vi "Adquisicion_6218.vi"() -> ()   [LabVIEW 2011]
uses:
  <vilib>/Utility/config.llb/Read Key (String).vi
  <vilib>/Utility/config.llb/Read Key (Double).vi
  <vilib>/Utility/config.llb/Write Key (String).vi
  <vilib>/Utility/config.llb/Write Key (Double).vi
  <vilib>/Utility/config.llb/NI_LVConfig.lvlib
  <vilib>/Analysis/NI_AALBase.lvlib
panel:
  out "Boolean 10":bool
  in  "Guardar":bool
  in  "Path2":bool
  in  "Datapath":bool
  in  "Path1":bool=TRUE
  in  "Tiempo":dbl
  in  "index 3":i32
  in  "index":i32
  out "reset3":bool
  out "reset2":bool
  out "reset":bool
  out "Time has Elapsed 2":bool caption="Time has Elapsed"
  out "Time has Elapsed":bool
  out "appended array":string[](array[string])
  in  "Tab Control 9":enum32{"Page 1", "Page 2", "Page 3"}(tab)
  in  "CH16":string="CH16"
  in  "CH15":string="CH15"
  in  "CH14":string="CH14"
  in  "CH13":string="CH13"
  in  "CH12":string="CH12"
  in  "CH11":string="CH11"
  in  "CH10":string="CH10"
  in  "CH9":string="CH9"
  in  "Tasa de Adquisicion":dbl=1000.0
  in  "CH8":string="CH8"
  in  "CH7":string="CH7"
  in  "CH6":string="CH6"
  in  "CH5":string="CH5"
  in  "CH4 2":string="CH4"
  in  "CH3":string="CH3"
  in  "CH2 2":string="CH2"
  in  "CH1":string="CH1"
  out "Voltaje":dbl
  out "Medida":dbl
  in  "m1":dbl
  in  "b1":dbl
  out "Voltaje":dbl
  in  "m2":dbl
  in  "b2":dbl
  out "Medida":dbl
  in  "m3":dbl
  in  "m4":dbl
  in  "b3":dbl
  in  "b4":dbl
  out "Voltaje":dbl
  out "Voltaje":dbl
  out "Medida":dbl
  out "Medida":dbl
  out "Medida":dbl
  in  "b5":dbl
  in  "m5":dbl
  out "Voltaje":dbl
  out "Medida":dbl
  in  "m6":dbl
  in  "b6":dbl
  out "Voltaje":dbl
  out "Medida":dbl
  in  "m7":dbl
  in  "b7":dbl
  out "Voltaje":dbl
  out "Voltaje":dbl
  in  "b8":dbl
  in  "m8":dbl
  out "Medida":dbl
  out "CH1":string
  out "CH2":string
  out "CH3":string
  out "CH4":string
  out "CH5":string
  out "CH6":string
  out "CH7":string
  out "CH8":string
  in  "Boolean":bool=TRUE
  in  "Boolean 2":bool=TRUE
  in  "Boolean 3":bool=TRUE
  in  "Boolean 4":bool=TRUE
  in  "Boolean 6":bool=TRUE
  in  "Boolean 5":bool=TRUE
  in  "Boolean 7":bool=TRUE
  in  "Boolean 8":bool=TRUE
  in  "Numero de Muestras":i32=1
  in  "file path":path=path "C:/Users/Zulueta/Documents/Pasantia/Mediciones"
  out "Tiempo":dbl caption="Elapsed Time (s)"
  in  "Iniciar":bool
  out "Boolean 9":bool
  in  "reset 2":bool caption="reset"
  out "q'":bool
  out "Tiempo":dbl caption="Elapsed Time (s)"
  in  "file path 2":path=path "C:/Users/Zulueta/Documents/Pasantia/Mediciones_Tiempo"
  out "Tiempo":dbl caption="Elapsed Time (s)"
  out "q2'":bool
  in  "?":bool
  in  "file path 3":path=path "C:/Users/Zulueta/Documents/Pasantia/Mediciones_Promedio"
  in  "Tiempo \nde adquisición":enum32{"Segundos", "Minutos", "Horas"}(tab) caption="Tiempo de adquisición"
  in  "?":dbl
  in  "?":dbl
  in  "?":dbl
  in  "stop":bool
  in  "Guardar Configuracion":bool
  in  "s":bool=TRUE
  in  "m9":dbl
  in  "b9":dbl
  out "s? t:f":dbl
  out "x+y":dbl
  in  "s 3":bool=TRUE
  out "s? t:f 2":dbl
  in  "m10":dbl
  in  "b10":dbl
  out "x+y 2":dbl
  out "s? t:f 3":dbl
  in  "m11":dbl
  in  "b11":dbl
  in  "s 6":bool=TRUE
  out "x+y 3":dbl
  in  "s 7":bool=TRUE
  out "s? t:f 4":dbl
  in  "m12":dbl
  in  "b12":dbl
  out "x+y 4":dbl
  in  "s 9":bool=TRUE
  in  "m13":dbl
  out "s? t:f 5":dbl
  in  "b13":dbl
  out "x+y 5":dbl
  in  "m14":dbl
  out "s? t:f 6":dbl
  in  "s 11":bool=TRUE
  in  "b14":dbl
  out "x+y 6":dbl
  in  "s 13":bool=TRUE
  out "s? t:f 7":dbl
  in  "m15":dbl
  in  "b15":dbl
  out "x+y 7":dbl
  in  "s 15":bool=TRUE
  in  "m16":dbl
  out "x+y 8":dbl
  out "s? t:f 8":dbl
  in  "b16":dbl
  out "CH9":string="CH8"
  out "CH10":string="CH10"
  out "CH11":string="CH11"
  out "CH12":string="CH12"
  out "CH13 3":string="CH13"
  out "CH14 3":string="CH14"
  out "CH15 3":string="CH15"
  out "CH16 3":string="CH16"
  out "Waveform Chart 17":dbl(graph)
  out "Waveform Chart 16":dbl(graph)
  out "Waveform Chart 15":dbl(graph)
  out "Waveform Chart 14":dbl(graph)
  out "Waveform Chart 13":dbl(graph)
  out "Waveform Chart 12":dbl(graph)
  out "Waveform Chart 11":dbl(graph)
  out "Waveform Chart 2":dbl(graph)
  out "Waveform Chart 10":dbl(graph)
  out "Waveform Chart 9":dbl(graph)
  out "Waveform Chart 8":dbl(graph)
  out "Waveform Chart 7":dbl(graph)
  out "Waveform Chart 6":dbl(graph)
  out "Waveform Chart 5":dbl(graph)
  out "Waveform Chart 4":dbl(graph)
  out "Waveform Chart 3":dbl(graph)
  out "CH1":string
  out "CH2":string
  out "CH3":string
  out "CH4":string
  out "CH5":string
  out "CH6":string
  out "CH7":string
  out "CH8":string
  in  "Boolean 18":bool=TRUE
  in  "Boolean 19":bool=TRUE
  in  "Boolean 20":bool=TRUE
  in  "Boolean 21":bool=TRUE
  in  "Boolean 22":bool=TRUE
  in  "Boolean 23":bool=TRUE
  in  "Boolean 24":bool=TRUE
  in  "Boolean 25":bool=TRUE
  in  "s 2":bool=TRUE
  in  "s 4":bool
  in  "s 5":bool
  in  "s 8":bool
  in  "s 10":bool
  in  "s 12":bool
  in  "s 14":bool
  in  "s 16":bool
  out "CH9 3":string="CH8"
  out "CH10 2":string="CH8"
  out "CH11 2":string="CH8"
  out "CH12 2":string="CH8"
  out "CH13 2":string="CH8"
  out "CH14 2":string="CH8"
  out "CH15 2":string="CH8"
  out "CH16 2":string="CH8"
  out "Waveform Chart":T1(graph)
  out "Time":dbl
  # "On/Off"
  # "Pendiente"
  # "Medida"
  # "Offset"
  # "Voltaje"
  # "Aquirir muestras por solicitud"
  # "Adquirir muestras por tiempo definido"
  # "Adquirir promedio de cada canal en un tiempo T"
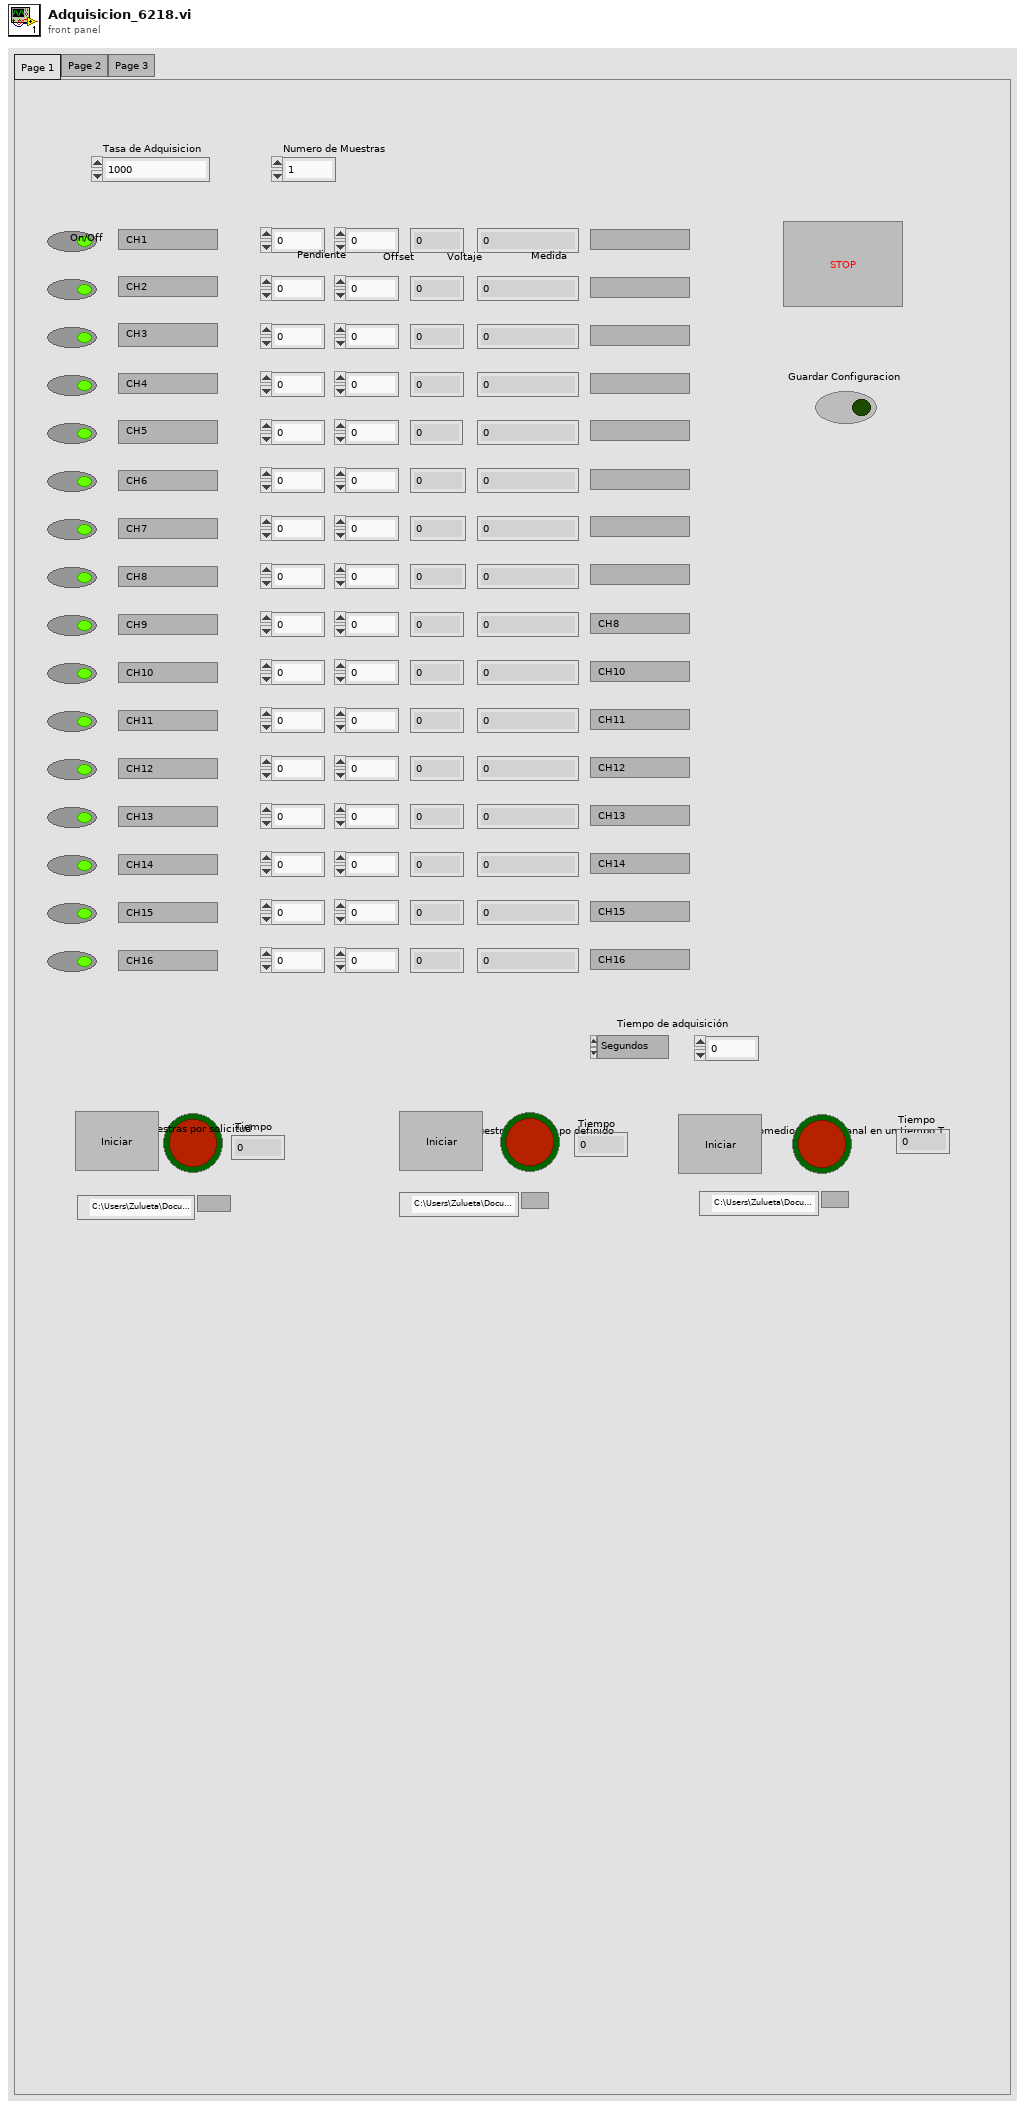
[diagram p1: front panel]
types:
  T1 = cluster{dbl, dbl, dbl, dbl, dbl, dbl, dbl, dbl, dbl, dbl, dbl, dbl, dbl, dbl, dbl, dbl}
  T2 = enum16{"big-endian, network order", "native, host order", "little-endian"}
  T3 = enum16{"open", "open or create", "create or replace", "create", "open (read-only)"}
  T4 = typedef "NI_LVConfig.lvlib/Config Data RefNum.ctl" = refnum<k1>
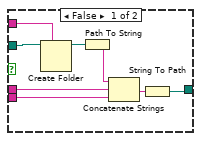
[diagram p2: hidden frame]
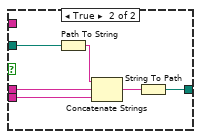
[diagram p3: hidden frame]
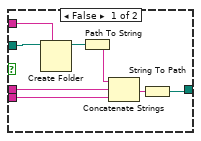
[diagram p4: hidden frame]
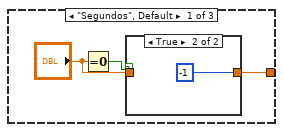
[diagram p11: hidden frame]
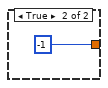
[diagram p13: hidden frame]
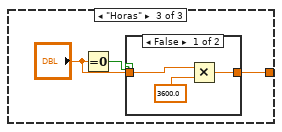
[diagram p14: hidden frame]
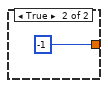
[diagram p15: hidden frame]
diagram:
  w177 = "_" ("replace string (\"\")")
  w178 = ":" ("search string")
  w110 = "\\" ("string")
  w156 = 0.0
  w6 = "Offsets" ("section")
  w44 = "Pendientes" ("section")
  w83 = TRUE ("read raw string? (F)")
  w74 = "Nombres_Canales" ("section")
  n1 = call <vilib>:"Open Config Data.vi"("configuration file path"=path "C:/Users/Zulueta/Documents/Pasantia/Configuracion_16Canales") -> ("error out"=w306:errorcluster, "refnum"=w307:T4)  [unwired: 8 in, 1 out]
  n2 = call-poly <vilib>:"Read Key.vi"("read raw string? (F)"=w83, "section"=w74, "error in (no error)"=w306, "key"="C1", "refnum"=w307) -> ("error out"=w302:errorcluster, "value"=w309:string, "refnum out"=w303:T4)  [unwired: 3 in, 1 out]
  n3 = property on="CH1" class="Str"("Value"=w309) -> ()  [unwired: 2 in, 2 out]
  n4 = call-poly <vilib>:"Read Key.vi"("read raw string? (F)"=w83, "section"=w74, "error in (no error)"=w302, "key"="C2", "refnum"=w303) -> ("error out"=w299:errorcluster, "value"=w304:string, "refnum out"=w298:T4)  [unwired: 3 in, 1 out]
  n5 = property on="CH2 2" class="Str"("Value"=w304) -> ()  [unwired: 2 in, 2 out]
  n6 = call-poly <vilib>:"Read Key.vi"("read raw string? (F)"=w83, "section"=w74, "error in (no error)"=w299, "key"="C3", "refnum"=w298) -> ("error out"=w295:errorcluster, "value"=w301:string, "refnum out"=w296:T4)  [unwired: 3 in, 1 out]
  n7 = property on="CH3" class="Str"("Value"=w301) -> ()  [unwired: 2 in, 2 out]
  n8 = call-poly <vilib>:"Read Key.vi"("read raw string? (F)"=w83, "section"=w74, "error in (no error)"=w295, "key"="C4", "refnum"=w296) -> ("error out"=w292:errorcluster, "value"=w297:string, "refnum out"=w293:T4)  [unwired: 3 in, 1 out]
  n9 = property on="CH4 2" class="Str"("Value"=w297) -> ()  [unwired: 2 in, 2 out]
  n10 = call-poly <vilib>:"Read Key.vi"("read raw string? (F)"=w83, "section"=w74, "error in (no error)"=w292, "key"="C5", "refnum"=w293) -> ("error out"=w287:errorcluster, "value"=w290:string, "refnum out"=w288:T4)  [unwired: 3 in, 1 out]
  n11 = property on="CH5" class="Str"("Value"=w290) -> ()  [unwired: 2 in, 2 out]
  n12 = call-poly <vilib>:"Read Key.vi"("read raw string? (F)"=w83, "section"=w74, "error in (no error)"=w287, "key"="C6", "refnum"=w288) -> ("error out"=w284:errorcluster, "value"=w289:string, "refnum out"=w285:T4)  [unwired: 3 in, 1 out]
  n13 = property on="CH6" class="Str"("Value"=w289) -> ()  [unwired: 2 in, 2 out]
  n14 = call-poly <vilib>:"Read Key.vi"("read raw string? (F)"=w83, "section"=w74, "error in (no error)"=w284, "key"="C7", "refnum"=w285) -> ("error out"=w279:errorcluster, "value"=w283:string, "refnum out"=w280:T4)  [unwired: 3 in, 1 out]
  n15 = property on="CH7" class="Str"("Value"=w283) -> ()  [unwired: 2 in, 2 out]
  n16 = call-poly <vilib>:"Read Key.vi"("read raw string? (F)"=w83, "section"=w74, "error in (no error)"=w279, "key"="C8", "refnum"=w280) -> ("error out"=w105:errorcluster, "value"=w281:string, "refnum out"=w106:T4)  [unwired: 3 in, 1 out]
  n17 = property on="CH8" class="Str"("Value"=w281) -> ()  [unwired: 2 in, 2 out]
  n18 = call-poly <vilib>:"Read Key.vi"("read raw string? (F)"=w83, "section"=w74, "error in (no error)"=w105, "key"="C9", "refnum"=w106) -> ("error out"=w101:errorcluster, "value"=w103:string, "refnum out"=w102:T4)  [unwired: 3 in, 1 out]
  n19 = property on="CH9" class="Str"("Value"=w103) -> ()  [unwired: 2 in, 2 out]
  n20 = call-poly <vilib>:"Read Key.vi"("read raw string? (F)"=w83, "section"=w74, "error in (no error)"=w101, "key"="C10", "refnum"=w102) -> ("error out"=w98:errorcluster, "value"=w97:string, "refnum out"=w99:T4)  [unwired: 3 in, 1 out]
  n21 = property on="CH10" class="Str"("Value"=w97) -> ()  [unwired: 2 in, 2 out]
  n22 = call-poly <vilib>:"Read Key.vi"("read raw string? (F)"=w83, "section"=w74, "error in (no error)"=w98, "key"="C11", "refnum"=w99) -> ("error out"=w93:errorcluster, "value"=w95:string, "refnum out"=w94:T4)  [unwired: 3 in, 1 out]
  n23 = property on="CH11" class="Str"("Value"=w95) -> ()  [unwired: 2 in, 2 out]
  n24 = call-poly <vilib>:"Read Key.vi"("read raw string? (F)"=w83, "section"=w74, "error in (no error)"=w93, "key"="C12", "refnum"=w94) -> ("error out"=w89:errorcluster, "value"=w91:string, "refnum out"=w90:T4)  [unwired: 3 in, 1 out]
  n25 = property on="CH12" class="Str"("Value"=w91) -> ()  [unwired: 2 in, 2 out]
  n26 = call-poly <vilib>:"Read Key.vi"("read raw string? (F)"=w83, "section"=w74, "error in (no error)"=w89, "key"="C13", "refnum"=w90) -> ("error out"=w86:errorcluster, "value"=w85:string, "refnum out"=w87:T4)  [unwired: 3 in, 1 out]
  n27 = property on="CH13" class="Str"("Value"=w85) -> ()  [unwired: 2 in, 2 out]
  n28 = call-poly <vilib>:"Read Key.vi"("read raw string? (F)"=w83, "section"=w74, "error in (no error)"=w86, "key"="C14", "refnum"=w87) -> ("error out"=w81:errorcluster, "value"=w79:string, "refnum out"=w82:T4)  [unwired: 3 in, 1 out]
  n29 = property on="CH14" class="Str"("Value"=w79) -> ()  [unwired: 2 in, 2 out]
  n30 = call-poly <vilib>:"Read Key.vi"("section"=w74, "error in (no error)"=w81, "key"="C15", "refnum"=w82) -> ("error out"=w77:errorcluster, "value"=w78:string, "refnum out"=w76:T4)  [unwired: 4 in, 1 out]
  n31 = Obtain Queue(name (unnamed)="CH9", element data type=w156) -> (queue out=w137:refnum<queue>)  [unwired: 3 in, 2 out]
  n32 = Obtain Queue(name (unnamed)="CH9(PSI)", element data type=w156) -> (queue out=w136:refnum<queue>)  [unwired: 3 in, 2 out]
  n33 = Obtain Queue(name (unnamed)="CH10", element data type=w156) -> (queue out=w135:refnum<queue>)  [unwired: 3 in, 2 out]
  n34 = Obtain Queue(name (unnamed)="CH1", element data type=w156) -> (queue out=w153:refnum<queue>)  [unwired: 3 in, 2 out]
  n35 = Obtain Queue(name (unnamed)="CH1(PSI)", element data type=w156) -> (queue out=w152:refnum<queue>)  [unwired: 3 in, 2 out]
  n36 = Obtain Queue(name (unnamed)="CH2", element data type=w156) -> (queue out=w151:refnum<queue>)  [unwired: 3 in, 2 out]
  n37 = Obtain Queue(name (unnamed)="CH2(PSI)", element data type=w156) -> (queue out=w150:refnum<queue>)  [unwired: 3 in, 2 out]
  n38 = Obtain Queue(name (unnamed)="CH3", element data type=w156) -> (queue out=w149:refnum<queue>)  [unwired: 3 in, 2 out]
  n39 = Obtain Queue(name (unnamed)="CH3(PSI)", element data type=w156) -> (queue out=w148:refnum<queue>)  [unwired: 3 in, 2 out]
  n40 = Obtain Queue(name (unnamed)="CH4", element data type=w156) -> (queue out=w147:refnum<queue>)  [unwired: 3 in, 2 out]
  n41 = Obtain Queue(name (unnamed)="CH4(PSI)", element data type=w156) -> (queue out=w146:refnum<queue>)  [unwired: 3 in, 2 out]
  n42 = Obtain Queue(name (unnamed)="CH5", element data type=w156) -> (queue out=w145:refnum<queue>)  [unwired: 3 in, 2 out]
  n43 = Obtain Queue(name (unnamed)="CH5(PSI)", element data type=w156) -> (queue out=w144:refnum<queue>)  [unwired: 3 in, 2 out]
  n44 = Obtain Queue(name (unnamed)="CH6", element data type=w156) -> (queue out=w143:refnum<queue>)  [unwired: 3 in, 2 out]
  n45 = Obtain Queue(name (unnamed)="CH6(PSI)", element data type=w156) -> (queue out=w142:refnum<queue>)  [unwired: 3 in, 2 out]
  n46 = Obtain Queue(name (unnamed)="CH7", element data type=w156) -> (queue out=w141:refnum<queue>)  [unwired: 3 in, 2 out]
  n47 = Obtain Queue(name (unnamed)="CH7(PSI)", element data type=w156) -> (queue out=w140:refnum<queue>)  [unwired: 3 in, 2 out]
  n48 = Obtain Queue(name (unnamed)="CH8", element data type=w156) -> (queue out=w139:refnum<queue>)  [unwired: 3 in, 2 out]
  n49 = Obtain Queue(name (unnamed)="CH8(PSI)", element data type=w156) -> (queue out=w138:refnum<queue>)  [unwired: 3 in, 2 out]
  n50 = Obtain Queue(name (unnamed)="CH10(PSI)", element data type=w156) -> (queue out=w134:refnum<queue>)  [unwired: 3 in, 2 out]
  n51 = Obtain Queue(name (unnamed)="CH11", element data type=w156) -> (queue out=w133:refnum<queue>)  [unwired: 3 in, 2 out]
  n52 = Obtain Queue(name (unnamed)="CH11(PSI)", element data type=w156) -> (queue out=w132:refnum<queue>)  [unwired: 3 in, 2 out]
  n53 = Obtain Queue(name (unnamed)="CH12", element data type=w156) -> (queue out=w131:refnum<queue>)  [unwired: 3 in, 2 out]
  n54 = Obtain Queue(name (unnamed)="CH12(PSI)", element data type=w156) -> (queue out=w130:refnum<queue>)  [unwired: 3 in, 2 out]
  n55 = Obtain Queue(name (unnamed)="CH13", element data type=w156) -> (queue out=w129:refnum<queue>)  [unwired: 3 in, 2 out]
  n56 = Obtain Queue(name (unnamed)="CH13(PSI)", element data type=w156) -> (queue out=w128:refnum<queue>)  [unwired: 3 in, 2 out]
  n57 = Obtain Queue(name (unnamed)="CH14", element data type=w156) -> (queue out=w127:refnum<queue>)  [unwired: 3 in, 2 out]
  n58 = Obtain Queue(name (unnamed)="CH14(PSI)", element data type=w156) -> (queue out=w126:refnum<queue>)  [unwired: 3 in, 2 out]
  n59 = Obtain Queue(name (unnamed)="CH15", element data type=w156) -> (queue out=w125:refnum<queue>)  [unwired: 3 in, 2 out]
  n60 = Obtain Queue(name (unnamed)="CH15(PSI)", element data type=w156) -> (queue out=w124:refnum<queue>)  [unwired: 3 in, 2 out]
  n61 = Obtain Queue(name (unnamed)="CH16", element data type=w156) -> (queue out=w123:refnum<queue>)  [unwired: 3 in, 2 out]
  n62 = Obtain Queue(name (unnamed)="CH16(PSI)", element data type=w156) -> (queue out=w122:refnum<queue>)  [unwired: 3 in, 2 out]
  n63 = property on="CH15" class="Str"("Value"=w78) -> ()  [unwired: 2 in, 2 out]
  n64 = call-poly <vilib>:"Read Key.vi"("section"=w74, "error in (no error)"=w77, "key"="C16", "refnum"=w76) -> ("error out"=w72:errorcluster, "value"=w71:string, "refnum out"=w73:T4)  [unwired: 4 in, 1 out]
  n65 = property on="CH16" class="Str"("Value"=w71) -> ()  [unwired: 2 in, 2 out]
  n66 = call-poly <vilib>:"Read Key.vi"("section"=w44, "error in (no error)"=w72, "key"="M1", "refnum"=w73) -> ("error out"=w274:errorcluster, "value"=w277:dbl, "refnum out"=w275:T4)  [unwired: 4 in, 1 out]
  n67 = property on="m1" class="DigNum (strict)"("Value"=w277) -> ()  [unwired: 2 in, 2 out]
  n68 = call-poly <vilib>:"Read Key.vi"("section"=w44, "error in (no error)"=w274, "key"="M2", "refnum"=w275) -> ("error out"=w270:errorcluster, "value"=w273:dbl, "refnum out"=w271:T4)  [unwired: 4 in, 1 out]
  n69 = property on="m2" class="DigNum (strict)"("Value"=w273) -> ()  [unwired: 2 in, 2 out]
  n70 = call-poly <vilib>:"Read Key.vi"("section"=w44, "error in (no error)"=w270, "key"="M3", "refnum"=w271) -> ("error out"=w267:errorcluster, "value"=w269:dbl, "refnum out"=w266:T4)  [unwired: 4 in, 1 out]
  n71 = property on="m3" class="DigNum (strict)"("Value"=w269) -> ()  [unwired: 2 in, 2 out]
  n72 = call-poly <vilib>:"Read Key.vi"("section"=w44, "error in (no error)"=w267, "key"="M4", "refnum"=w266) -> ("error out"=w263:errorcluster, "value"=w265:dbl, "refnum out"=w262:T4)  [unwired: 4 in, 1 out]
  n73 = property on="m4" class="DigNum (strict)"("Value"=w265) -> ()  [unwired: 2 in, 2 out]
  n74 = call-poly <vilib>:"Read Key.vi"("section"=w44, "error in (no error)"=w263, "key"="M5", "refnum"=w262) -> ("error out"=w259:errorcluster, "value"=w261:dbl, "refnum out"=w258:T4)  [unwired: 4 in, 1 out]
  n75 = property on="m5" class="DigNum (strict)"("Value"=w261) -> ()  [unwired: 2 in, 2 out]
  n76 = call-poly <vilib>:"Read Key.vi"("section"=w44, "error in (no error)"=w259, "key"="M6", "refnum"=w258) -> ("error out"=w254:errorcluster, "value"=w257:dbl, "refnum out"=w255:T4)  [unwired: 4 in, 1 out]
  n77 = property on="m6" class="DigNum (strict)"("Value"=w257) -> ()  [unwired: 2 in, 2 out]
  n78 = call-poly <vilib>:"Read Key.vi"("section"=w44, "error in (no error)"=w254, "key"="M7", "refnum"=w255) -> ("error out"=w251:errorcluster, "value"=w253:dbl, "refnum out"=w250:T4)  [unwired: 4 in, 1 out]
  n79 = property on="m7" class="DigNum (strict)"("Value"=w253) -> ()  [unwired: 2 in, 2 out]
  n80 = while {
    tunnel: w153 -> [w421]
    tunnel: w151 -> [w516]
    tunnel: w149 -> [w515]
    tunnel: w147 -> [w514]
    tunnel: w145 -> [w513]
    tunnel: w143 -> [w512]
    tunnel: w141 -> [w511]
    tunnel: w139 -> [w510]
    tunnel: w152 -> [w506]
    tunnel: w150 -> [w501]
    tunnel: w148 -> [w500]
    tunnel: w146 -> [w495]
    tunnel: w142 -> [w485]
    tunnel: w144 -> [w490]
    tunnel: w140 -> [w484]
    tunnel: w138 -> [w483]
    shift-right: [w420] -> _
    shift-left: w156 -> [w320]
    tunnel: w137 -> [w414]
    tunnel: w136 -> [w406]
    tunnel: w135 -> [w402]
    tunnel: w134 -> [w394]
    tunnel: w133 -> [w390]
    tunnel: w132 -> [w387]
    tunnel: w131 -> [w378]
    tunnel: w130 -> [w377]
    tunnel: w129 -> [w367]
    tunnel: w128 -> [w365]
    tunnel: w127 -> [w355]
    tunnel: w126 -> [w354]
    tunnel: w125 -> [w342]
    tunnel: w124 -> [w341]
    tunnel: w123 -> [w330]
    tunnel: w122 -> [w328]
    stop <- "stop" stop-if-true
    w329 = 0.0 ("f")
    n81 = call "DAQ Assistant"("rate"="Tasa de Adquisicion", "number of samples"="Numero de Muestras") -> ("data"=w417:dynamicdata, "error out"=w418:errorcluster)  [unwired: 14 in, 2 out]
    n82 = call <vilib>:"Clear Errors.vi"("error in (no error)"=w418) -> ()  [unwired: 6 in, 1 out]
    n83 = Split Signals(w417) -> (w469:dynamicdata, w504:dynamicdata, w499:dynamicdata, w494:dynamicdata, w489:dynamicdata, w482:dynamicdata, w478:dynamicdata, w474:dynamicdata, w411:dynamicdata, w401:dynamicdata, w381:dynamicdata, w375:dynamicdata, w352:dynamicdata, w338:dynamicdata, w339:dynamicdata, w326:dynamicdata)  [unwired: 16 in]
    n84 = call "Convert from Dynamic Data"("Dynamic Data Type"=w469) -> ("Scalar"=w458:dbl)  [unwired: 3 in]
    n85 = call "Convert from Dynamic Data2"("Dynamic Data Type"=w504) -> ("Scalar"=w468:dbl)  [unwired: 3 in]
    n86 = call "Convert from Dynamic Data3"("Dynamic Data Type"=w499) -> ("Scalar"=w466:dbl)  [unwired: 3 in]
    n87 = call "Convert from Dynamic Data4"("Dynamic Data Type"=w494) -> ("Scalar"=w464:dbl)  [unwired: 3 in]
    n88 = call "Convert from Dynamic Data5"("Dynamic Data Type"=w489) -> ("Scalar"=w462:dbl)  [unwired: 3 in]
    n89 = Select(t=w458, s="Boolean", f=w329) -> (s? t:f=w457:dbl)
    "Voltaje" <- w457
    n90 = call "Convert from Dynamic Data6"("Dynamic Data Type"=w482) -> ("Scalar"=w460:dbl)  [unwired: 3 in]
    n91 = call "Convert from Dynamic Data7"("Dynamic Data Type"=w478) -> ("Scalar"=w450:dbl)  [unwired: 3 in]
    n92 = call "Convert from Dynamic Data11"("Dynamic Data Type"=w381) -> ("Scalar"=w382:dbl)  [unwired: 3 in]
    n93 = call "Convert from Dynamic Data12"("Dynamic Data Type"=w375) -> ("Scalar"=w376:dbl)  [unwired: 3 in]
    n94 = call "Convert from Dynamic Data13"("Dynamic Data Type"=w352) -> ("Scalar"=w364:dbl)  [unwired: 3 in]
    n95 = call "Convert from Dynamic Data14"("Dynamic Data Type"=w338) -> ("Scalar"=w353:dbl)  [unwired: 3 in]
    n96 = call "Convert from Dynamic Data9"("Dynamic Data Type"=w411) -> ("Scalar"=w412:dbl)  [unwired: 3 in]
    n97 = call "Convert from Dynamic Data10"("Dynamic Data Type"=w401) -> ("Scalar"=w400:dbl)  [unwired: 3 in]
    n98 = call "Convert from Dynamic Data15"("Dynamic Data Type"=w339) -> ("Scalar"=w340:dbl)  [unwired: 3 in]
    n99 = Select(t=w468, s="Boolean 2", f=w329) -> (s? t:f=w456:dbl)
    "Voltaje" <- w456
    n100 = call "Convert from Dynamic Data8"("Dynamic Data Type"=w474) -> ("Scalar"=w448:dbl)  [unwired: 3 in]
    n101 = call "Convert from Dynamic Data16"("Dynamic Data Type"=w326) -> ("Scalar"=w327:dbl)  [unwired: 3 in]
    n102 = Select(t=w466, s="Boolean 3", f=w329) -> (s? t:f=w455:dbl)
    "Voltaje" <- w455
    n103 = Select(t=w464, s="Boolean 4", f=w329) -> (s? t:f=w454:dbl)
    "Voltaje" <- w454
    n104 = Enqueue Element(queue=w421, element=w469) -> ()  [unwired: 2 in, 3 out]
    n105 = Enqueue Element(queue=w516, element=w504) -> ()  [unwired: 2 in, 3 out]
    n106 = Enqueue Element(queue=w515, element=w499) -> ()  [unwired: 2 in, 3 out]
    n107 = Enqueue Element(queue=w514, element=w494) -> ()  [unwired: 2 in, 3 out]
    n108 = Enqueue Element(queue=w513, element=w489) -> ()  [unwired: 2 in, 3 out]
    n109 = Enqueue Element(queue=w512, element=w482) -> ()  [unwired: 2 in, 3 out]
    n110 = Enqueue Element(queue=w511, element=w478) -> ()  [unwired: 2 in, 3 out]
    n111 = Enqueue Element(queue=w510, element=w474) -> ()  [unwired: 2 in, 3 out]
    n112 = Enqueue Element(queue=w414, element=w411) -> ()  [unwired: 2 in, 3 out]
    n113 = Select(t=w462, s="Boolean 5", f=w329) -> (s? t:f=w453:dbl)
    "Voltaje" <- w453
    n114 = Enqueue Element(queue=w402, element=w401) -> ()  [unwired: 2 in, 3 out]
    n115 = Enqueue Element(queue=w390, element=w381) -> ()  [unwired: 2 in, 3 out]
    n116 = Enqueue Element(queue=w378, element=w375) -> ()  [unwired: 2 in, 3 out]
    n117 = Enqueue Element(queue=w367, element=w352) -> ()  [unwired: 2 in, 3 out]
    n118 = Enqueue Element(queue=w355, element=w338) -> ()  [unwired: 2 in, 3 out]
    n119 = Select(t=w450, s="Boolean 7", f=w329) -> (s? t:f=w449:dbl)
    "Voltaje" <- w449
    n120 = Enqueue Element(queue=w342, element=w339) -> ()  [unwired: 2 in, 3 out]
    n121 = Enqueue Element(queue=w330, element=w326) -> ()  [unwired: 2 in, 3 out]
    n122 = Select(t=w460, s="Boolean 6", f=w329) -> (s? t:f=w452:dbl)
    "Voltaje" <- w452
    n123 = Select(t=w400, s="s 3", f=w329) -> (s? t:f=w398:dbl)
    "s? t:f 2" <- w398
    n124 = Select(t=w448, s="Boolean 8", f=w329) -> (s? t:f=w447:dbl)
    "Voltaje" <- w447
    n125 = Select(t=w412, s="s", f=w329) -> (s? t:f=w410:dbl)
    "s? t:f" <- w410
    n126 = Select(t=w382, s="s 6", f=w329) -> (s? t:f=w388:dbl)
    "s? t:f 3" <- w388
    n127 = Select(t=w376, s="s 7", f=w329) -> (s? t:f=w372:dbl)
    "s? t:f 4" <- w372
    n128 = Select(t=w364, s="s 9", f=w329) -> (s? t:f=w362:dbl)
    "s? t:f 5" <- w362
    n129 = Select(t=w353, s="s 11", f=w329) -> (s? t:f=w351:dbl)
    "s? t:f 6" <- w351
    n130 = Select(t=w340, s="s 13", f=w329) -> (s? t:f=w336:dbl)
    "s? t:f 7" <- w336
    n131 = Select(t=w327, s="s 15", f=w329) -> (s? t:f=w324:dbl)
    "s? t:f 8" <- w324
    n132 = Multiply(x=w457, y="m1") -> (x*y=w508:dbl)
    n133 = Multiply(x=w456, y="m2") -> (x*y=w503:dbl)
    n134 = Multiply(x=w455, y="m3") -> (x*y=w497:dbl)
    n135 = Multiply(x=w454, y="m4") -> (x*y=w492:dbl)
    n136 = Multiply(x=w453, y="m5") -> (x*y=w487:dbl)
    n137 = Multiply(x=w449, y="m7") -> (x*y=w476:dbl)
    n138 = Multiply(x=w452, y="m6") -> (x*y=w480:dbl)
    n139 = Multiply(x=w410, y="m9") -> (x*y=w409:dbl)
    n140 = Multiply(x=w447, y="m8") -> (x*y=w472:dbl)
    n141 = Multiply(x=w336, y="m15") -> (x*y=w335:dbl)
    n142 = Multiply(x=w324, y="m16") -> (x*y=w323:dbl)
    n143 = Multiply(x=w398, y="m10") -> (x*y=w397:dbl)
    n144 = Multiply(x=w388, y="m11") -> (x*y=w389:dbl)
    n145 = Multiply(x=w372, y="m12") -> (x*y=w373:dbl)
    n146 = Multiply(x=w362, y="m13") -> (x*y=w360:dbl)
    n147 = Multiply(x=w351, y="m14") -> (x*y=w348:dbl)
    n148 = Add(x=w508, y="b1") -> (x+y=w437:dbl)
    "Waveform Chart 10" <- w437
    "Medida" <- w437
    n149 = Add(x=w503, y="b2") -> (x+y=w436:dbl)
    "Waveform Chart 3" <- w436
    "Medida" <- w436
    n150 = Add(x=w409, y="b9") -> (x+y=w404:dbl)
    "x+y" <- w404
    "Waveform Chart 2" <- w404
    n151 = Add(x=w497, y="b3") -> (x+y=w435:dbl)
    "Waveform Chart 4" <- w435
    "Medida" <- w435
    n152 = Add(x=w492, y="b4") -> (x+y=w434:dbl)
    "Waveform Chart 5" <- w434
    "Medida" <- w434
    n153 = Add(x=w487, y="b5") -> (x+y=w433:dbl)
    "Waveform Chart 6" <- w433
    "Medida" <- w433
    n154 = Add(x=w480, y="b6") -> (x+y=w432:dbl)
    "Waveform Chart 7" <- w432
    "Medida" <- w432
    n155 = Add(x=w476, y="b7") -> (x+y=w431:dbl)
    "Waveform Chart 8" <- w431
    "Medida" <- w431
    n156 = Add(x=w472, y="b8") -> (x+y=w430:dbl)
    "Waveform Chart 9" <- w430
    "Medida" <- w430
    n157 = Add(x=w397, y="b10") -> (x+y=w393:dbl)
    "x+y 2" <- w393
    "Waveform Chart 11" <- w393
    n158 = Add(x=w389, y="b11") -> (x+y=w383:dbl)
    "x+y 3" <- w383
    "Waveform Chart 12" <- w383
    n159 = Add(x=w373, y="b12") -> (x+y=w369:dbl)
    "x+y 4" <- w369
    "Waveform Chart 13" <- w369
    n160 = Add(x=w360, y="b13") -> (x+y=w358:dbl)
    "x+y 5" <- w358
    "Waveform Chart 14" <- w358
    n161 = Add(x=w348, y="b14") -> (x+y=w346:dbl)
    "x+y 6" <- w346
    "Waveform Chart 15" <- w346
    n162 = Add(x=w335, y="b15") -> (x+y=w332:dbl)
    "x+y 7" <- w332
    "Waveform Chart 16" <- w332
    n163 = Add(x=w323, y="b16") -> (x+y=w316:dbl)
    "x+y 8" <- w316
    "Waveform Chart 17" <- w316
    n164 = Enqueue Element(queue=w483, element=w430) -> ()  [unwired: 2 in, 3 out]
    n165 = Enqueue Element(queue=w406, element=w404) -> ()  [unwired: 2 in, 3 out]
    n166 = Enqueue Element(queue=w354, element=w346) -> ()  [unwired: 2 in, 3 out]
    n167 = Enqueue Element(queue=w341, element=w332) -> ()  [unwired: 2 in, 3 out]
    n168 = Enqueue Element(queue=w328, element=w316) -> ()  [unwired: 2 in, 3 out]
    n169 = Enqueue Element(queue=w394, element=w393) -> ()  [unwired: 2 in, 3 out]
    n170 = Enqueue Element(queue=w387, element=w383) -> ()  [unwired: 2 in, 3 out]
    n171 = Enqueue Element(queue=w377, element=w369) -> ()  [unwired: 2 in, 3 out]
    n172 = Enqueue Element(queue=w365, element=w358) -> ()  [unwired: 2 in, 3 out]
    n173 = Enqueue Element(queue=w506, element=w437) -> ()  [unwired: 2 in, 3 out]
    n174 = Enqueue Element(queue=w501, element=w436) -> ()  [unwired: 2 in, 3 out]
    n175 = Enqueue Element(queue=w500, element=w435) -> ()  [unwired: 2 in, 3 out]
    n176 = Enqueue Element(queue=w495, element=w434) -> ()  [unwired: 2 in, 3 out]
    n177 = Enqueue Element(queue=w490, element=w433) -> ()  [unwired: 2 in, 3 out]
    n178 = Enqueue Element(queue=w485, element=w432) -> ()  [unwired: 2 in, 3 out]
    n179 = Enqueue Element(queue=w484, element=w431) -> ()  [unwired: 2 in, 3 out]
    n180 = Select(t=w437, s="Boolean 25", f=w320) -> (s? t:f=w429:dbl)
    n181 = Select(t=w436, s="Boolean 24", f=w320) -> (s? t:f=w428:dbl)
    n182 = Select(t=w435, s="Boolean 23", f=w320) -> (s? t:f=w427:dbl)
    n183 = Select(t=w434, s="Boolean 22", f=w320) -> (s? t:f=w426:dbl)
    n184 = Select(t=w433, s="Boolean 21", f=w320) -> (s? t:f=w425:dbl)
    n185 = Select(t=w432, s="Boolean 20", f=w320) -> (s? t:f=w424:dbl)
    n186 = Select(t=w431, s="Boolean 19", f=w320) -> (s? t:f=w423:dbl)
    n187 = Select(t=w430, s="Boolean 18", f=w320) -> (s? t:f=w422:dbl)
    n188 = Select(t=w404, s="s 2", f=w320) -> (s? t:f=w405:dbl)
    n189 = Select(t=w393, s="s 4", f=w320) -> (s? t:f=w392:dbl)
    n190 = Select(t=w383, s="s 5", f=w320) -> (s? t:f=w384:dbl)
    n191 = Select(t=w369, s="s 8", f=w320) -> (s? t:f=w368:dbl)
    n192 = Select(t=w358, s="s 10", f=w320) -> (s? t:f=w356:dbl)
    n193 = Select(t=w346, s="s 12", f=w320) -> (s? t:f=w344:dbl)
    n194 = Select(t=w332, s="s 14", f=w320) -> (s? t:f=w343:dbl)
    n195 = Select(t=w316, s="s 16", f=w320) -> (s? t:f=w319:dbl)
    n196 = Bundle(w429, w428, w427, w426, w425, w424, w423, w422, w405, w392, w384, w368, w356, w344, w343, w319) -> (w318:T1)  [unwired: 1 in]
    "Waveform Chart" <- w318
    n197 = Cluster To Array(cluster=w318) -> (array=w317:dbl[])
    n198 = call <vilib>:"Mean.vi"("X"=w317) -> ("mean"=w420:dbl)  [unwired: 1 out]
    "Boolean 10" <- "stop"
  }
  n199 = call-poly <vilib>:"Read Key.vi"("section"=w44, "error in (no error)"=w251, "key"="M8", "refnum"=w250) -> ("error out"=w69:errorcluster, "value"=w249:dbl, "refnum out"=w70:T4)  [unwired: 4 in, 1 out]
  n200 = property on="m8" class="DigNum (strict)"("Value"=w249) -> ()  [unwired: 2 in, 2 out]
  n201 = Get Date/Time In Seconds() -> (seconds since 1Jan1904=w189:timestamp)
  n202 = call-poly <vilib>:"Read Key.vi"("section"=w44, "error in (no error)"=w69, "key"="M9", "refnum"=w70) -> ("error out"=w66:errorcluster, "value"=w64:dbl, "refnum out"=w65:T4)  [unwired: 4 in, 1 out]
  n203 = property on="m9" class="DigNum (strict)"("Value"=w64) -> ()  [unwired: 2 in, 2 out]
  n204 = call-poly <vilib>:"Read Key.vi"("section"=w44, "error in (no error)"=w66, "key"="M10", "refnum"=w65) -> ("error out"=w62:errorcluster, "value"=w60:dbl, "refnum out"=w63:T4)  [unwired: 4 in, 1 out]
  n205 = property on="m10" class="DigNum (strict)"("Value"=w60) -> ()  [unwired: 2 in, 2 out]
  n206 = Get Date/Time String(date format (0)=enum16{"short", "long", "abbreviated"}."abbreviated", seconds (now)=w189, want seconds? (F)=TRUE) -> (date string=w111:string, time string=w179:string)
  n207 = Path To String(path="file path") -> (string=w193:string)
  n208 = Path To String(path="file path 2") -> (string=w185:string)
  n209 = Path To String(path="file path 3") -> (string=w181:string)
  n210 = call-poly <vilib>:"Read Key.vi"("section"=w44, "error in (no error)"=w62, "key"="M11", "refnum"=w63) -> ("error out"=w59:errorcluster, "value"=w56:dbl, "refnum out"=w58:T4)  [unwired: 4 in, 1 out]
  n211 = property on="m11" class="DigNum (strict)"("Value"=w56) -> ()  [unwired: 2 in, 2 out]
  n212 = call-poly <vilib>:"Read Key.vi"("section"=w44, "error in (no error)"=w59, "key"="M12", "refnum"=w58) -> ("error out"=w54:errorcluster, "value"=w43:dbl, "refnum out"=w55:T4)  [unwired: 4 in, 1 out]
  n213 = Concatenate Strings(w193, w110, w111) -> (w191:string)
  n214 = Concatenate Strings(w185, w110, w111) -> (w186:string)
  n215 = Concatenate Strings(w181, w110, w111) -> (w180:string)
  n216 = property on="m12" class="DigNum (strict)"("Value"=w43) -> ()  [unwired: 2 in, 2 out]
  n217 = call-poly <vilib>:"Read Key.vi"("section"=w44, "error in (no error)"=w54, "key"="M13", "refnum"=w55) -> ("error out"=w51:errorcluster, "value"=w42:dbl, "refnum out"=w50:T4)  [unwired: 4 in, 1 out]
  n218 = property on="m13" class="DigNum (strict)"("Value"=w42) -> ()  [unwired: 2 in, 2 out]
  n219 = String To Path(string=w191) -> (path=w192:path)
  n220 = String To Path(string=w186) -> (path=w187:path)
  n221 = String To Path(string=w180) -> (path=w176:path)
  n222 = Search and Replace String(replace all?=TRUE ("replace all? (F)"), input string=w179, search string=w178, replace string=w177) -> (result string=w120:string)  [unwired: 4 in, 3 out]
  n223 = Search and Replace String(replace all?=TRUE ("replace all? (F)"), input string=w179, search string=w178, replace string=w177) -> (result string=w114:string)  [unwired: 4 in, 3 out]
  n224 = Search and Replace String(replace all?=TRUE ("replace all? (F)"), input string=w179, search string=w178, replace string=w177) -> (result string=w109:string)  [unwired: 4 in, 3 out]
  n225 = call-poly <vilib>:"Read Key.vi"("section"=w44, "error in (no error)"=w51, "key"="M14", "refnum"=w50) -> ("error out"=w48:errorcluster, "value"=w41:dbl, "refnum out"=w47:T4)  [unwired: 4 in, 1 out]
  n226 = property on="m14" class="DigNum (strict)"("Value"=w41) -> ()  [unwired: 2 in, 2 out]
  n227 = call-poly <vilib>:"Read Key.vi"("section"=w44, "error in (no error)"=w48, "key"="M15", "refnum"=w47) -> ("error out"=w45:errorcluster, "value"=w39:dbl, "refnum out"=w46:T4)  [unwired: 4 in, 1 out]
  n228 = call <vilib>:"Check if File or Folder Exists.vi"("path"=w192) -> ("file or folder exists?"=w118:bool, "dup path"=w121:path)  [unwired: 8 in, 1 out]
  n229 = call <vilib>:"Check if File or Folder Exists.vi"("path"=w187) -> ("file or folder exists?"=w117:bool, "dup path"=w116:path)  [unwired: 8 in, 1 out]
  n230 = call <vilib>:"Check if File or Folder Exists.vi"("path"=w176) -> ("file or folder exists?"=w113:bool, "dup path"=w112:path)  [unwired: 8 in, 1 out]
  n231 = property on="m15" class="DigNum (strict)"("Value"=w39) -> ()  [unwired: 2 in, 2 out]
  n232 = call-poly <vilib>:"Read Key.vi"("section"=w44, "error in (no error)"=w45, "key"="M16", "refnum"=w46) -> ("error out"=w36:errorcluster, "value"=w38:dbl, "refnum out"=w37:T4)  [unwired: 4 in, 1 out]
  n233 = property on="m16" class="DigNum (strict)"("Value"=w38) -> ()  [unwired: 2 in, 2 out]
  n234 = case shown="False" w117 {
    tunnel: w116 -> [w523 w530]
    tunnel: w110 -> [w521 w527]
    tunnel: w114 -> [w520 w526]
    tunnel: [w518 w525] -> w115
    tunnel: w111 -> [w517 _]
    frame False {
      n235 = Create Folder(prompt (Create Folder)=w517, path (use dialog)=w523) -> (created path=w524:path)  [unwired: 1 in, 2 out]
      n236 = Path To String(path=w524) -> (string=w522:string)
      n237 = Concatenate Strings(w522, w521, w520) -> (w519:string)
      n238 = String To Path(string=w519) -> (path=w518:path)
    }
    frame True {
      n239 = Path To String(path=w530) -> (string=w528:string)
      n240 = Concatenate Strings(w528, w527, w526) -> (w529:string)
      n241 = String To Path(string=w529) -> (path=w525:path)
    }
  }
  n242 = case shown="True" w118 {
    tunnel: w121 -> [w537 w544]
    tunnel: w110 -> [w535 w541]
    tunnel: w120 -> [w534 w540]
    tunnel: [w532 w539] -> w119
    tunnel: w111 -> [w531 _]
    frame False {
      n243 = Create Folder(prompt (Create Folder)=w531, path (use dialog)=w537) -> (created path=w538:path)  [unwired: 1 in, 2 out]
      n244 = Path To String(path=w538) -> (string=w536:string)
      n245 = Concatenate Strings(w536, w535, w534) -> (w533:string)
      n246 = String To Path(string=w533) -> (path=w532:path)
    }
    frame True {
      n247 = Path To String(path=w544) -> (string=w542:string)
      n248 = Concatenate Strings(w542, w541, w540) -> (w543:string)
      n249 = String To Path(string=w543) -> (path=w539:path)
    }
  }
  n250 = case shown="True" w113 {
    tunnel: w112 -> [w551 w558]
    tunnel: w110 -> [w549 w555]
    tunnel: w109 -> [w548 w554]
    tunnel: [w546 w553] -> w108
    tunnel: w111 -> [w545 _]
    frame False {
      n251 = Create Folder(prompt (Create Folder)=w545, path (use dialog)=w551) -> (created path=w552:path)  [unwired: 1 in, 2 out]
      n252 = Path To String(path=w552) -> (string=w550:string)
      n253 = Concatenate Strings(w550, w549, w548) -> (w547:string)
      n254 = String To Path(string=w547) -> (path=w546:path)
    }
    frame True {
      n255 = Path To String(path=w558) -> (string=w556:string)
      n256 = Concatenate Strings(w556, w555, w554) -> (w557:string)
      n257 = String To Path(string=w557) -> (path=w553:path)
    }
  }
  n258 = call-poly <vilib>:"Read Key.vi"("section"=w6, "error in (no error)"=w36, "key"="B1", "refnum"=w37) -> ("error out"=w245:errorcluster, "value"=w247:dbl, "refnum out"=w244:T4)  [unwired: 4 in, 1 out]
  n259 = property on="b1" class="DigNum (strict)"("Value"=w247) -> ()  [unwired: 2 in, 2 out]
  n260 = call-poly <vilib>:"Read Key.vi"("section"=w6, "error in (no error)"=w245, "key"="B2", "refnum"=w244) -> ("error out"=w241:errorcluster, "value"=w243:dbl, "refnum out"=w240:T4)  [unwired: 4 in, 1 out]
  n261 = property on="b2" class="DigNum (strict)"("Value"=w243) -> ()  [unwired: 2 in, 2 out]
  n262 = call-poly <vilib>:"Read Key.vi"("section"=w6, "error in (no error)"=w241, "key"="B3", "refnum"=w240) -> ("error out"=w237:errorcluster, "value"=w239:dbl, "refnum out"=w236:T4)  [unwired: 4 in, 1 out]
  n263 = property on="b3" class="DigNum (strict)"("Value"=w239) -> ()  [unwired: 2 in, 2 out]
  n264 = call-poly <vilib>:"Read Key.vi"("section"=w6, "error in (no error)"=w237, "key"="B4", "refnum"=w236) -> ("error out"=w232:errorcluster, "value"=w235:dbl, "refnum out"=w233:T4)  [unwired: 4 in, 1 out]
  n265 = property on="b4" class="DigNum (strict)"("Value"=w235) -> ()  [unwired: 2 in, 2 out]
  n266 = call-poly <vilib>:"Read Key.vi"("section"=w6, "error in (no error)"=w232, "key"="B5", "refnum"=w233) -> ("error out"=w229:errorcluster, "value"=w231:dbl, "refnum out"=w228:T4)  [unwired: 4 in, 1 out]
  n267 = property on="b5" class="DigNum (strict)"("Value"=w231) -> ()  [unwired: 2 in, 2 out]
  n268 = call-poly <vilib>:"Read Key.vi"("section"=w6, "error in (no error)"=w229, "key"="B6", "refnum"=w228) -> ("error out"=w224:errorcluster, "value"=w227:dbl, "refnum out"=w225:T4)  [unwired: 4 in, 1 out]
  n269 = property on="b6" class="DigNum (strict)"("Value"=w227) -> ()  [unwired: 2 in, 2 out]
  n270 = call-poly <vilib>:"Read Key.vi"("section"=w6, "error in (no error)"=w224, "key"="B7", "refnum"=w225) -> ("error out"=w220:errorcluster, "value"=w223:dbl, "refnum out"=w221:T4)  [unwired: 4 in, 1 out]
  n271 = property on="b7" class="DigNum (strict)"("Value"=w223) -> ()  [unwired: 2 in, 2 out]
  n272 = call-poly <vilib>:"Read Key.vi"("section"=w6, "error in (no error)"=w220, "key"="B8", "refnum"=w221) -> ("error out"=w34:errorcluster, "value"=w219:dbl, "refnum out"=w35:T4)  [unwired: 4 in, 1 out]
  n273 = property on="b8" class="DigNum (strict)"("Value"=w219) -> ()  [unwired: 2 in, 2 out]
  n274 = call-poly <vilib>:"Read Key.vi"("section"=w6, "error in (no error)"=w34, "key"="B9", "refnum"=w35) -> ("error out"=w30:errorcluster, "value"=w26:dbl, "refnum out"=w31:T4)  [unwired: 4 in, 1 out]
  n275 = property on="b9" class="DigNum (strict)"("Value"=w26) -> ()  [unwired: 2 in, 2 out]
  n276 = call-poly <vilib>:"Read Key.vi"("section"=w6, "error in (no error)"=w30, "key"="B10", "refnum"=w31) -> ("error out"=w28:errorcluster, "value"=w25:dbl, "refnum out"=w27:T4)  [unwired: 4 in, 1 out]
  n277 = property on="b10" class="DigNum (strict)"("Value"=w25) -> ()  [unwired: 2 in, 2 out]
  n278 = call-poly <vilib>:"Read Key.vi"("section"=w6, "error in (no error)"=w28, "key"="B11", "refnum"=w27) -> ("error out"=w22:errorcluster, "value"=w24:dbl, "refnum out"=w23:T4)  [unwired: 4 in, 1 out]
  n279 = TDMS Open(6:TRUE ("disable buffering? (T)"), 7:enum16{"1.0", "2.0"}."2.0" ("file format version (2.0)"), 9:T2."little-endian" ("byte order (2:little-endian)"), 10:T3."open or create" ("operation (0:open)"), 11:w119) -> (3:w196:refnum<k34>)  [unwired: 1 in, 1 out]
  n280 = TDMS Open(6:TRUE ("disable buffering? (T)"), 7:enum16{"1.0", "2.0"}."2.0" ("file format version (2.0)"), 9:T2."little-endian" ("byte order (2:little-endian)"), 10:T3."open or create" ("operation (0:open)"), 11:w108) -> (3:w171:refnum<k34>)  [unwired: 1 in, 1 out]
  n281 = property on="b11" class="DigNum (strict)"("Value"=w24) -> ()  [unwired: 2 in, 2 out]
  n282 = TDMS Open(6:TRUE ("disable buffering? (T)"), 7:enum16{"1.0", "2.0"}."2.0" ("file format version (2.0)"), 9:T2."little-endian" ("byte order (2:little-endian)"), 10:T3."open or create" ("operation (0:open)"), 11:w115) -> (3:w195:refnum<k34>)  [unwired: 1 in, 1 out]
  n283 = call-poly <vilib>:"Read Key.vi"("section"=w6, "error in (no error)"=w22, "key"="B12", "refnum"=w23) -> ("error out"=w20:errorcluster, "value"=w15:dbl, "refnum out"=w19:T4)  [unwired: 4 in, 1 out]
  n284 = property on="b12" class="DigNum (strict)"("Value"=w15) -> ()  [unwired: 2 in, 2 out]
  n285 = call-poly <vilib>:"Read Key.vi"("section"=w6, "error in (no error)"=w20, "key"="B13", "refnum"=w19) -> ("error out"=w16:errorcluster, "value"=w14:dbl, "refnum out"=w17:T4)  [unwired: 4 in, 1 out]
  n286 = while {
    tunnel: w196 -> [w686]
    tunnel: w195 -> [w685]
    tunnel: w171 -> [w676]
    tunnel: w153 -> [w610]
    tunnel: w152 -> [w624]
    tunnel: w151 -> [w609]
    tunnel: w150 -> [w623]
    tunnel: w149 -> [w608]
    tunnel: w148 -> [w622]
    tunnel: w147 -> [w607]
    tunnel: w146 -> [w621]
    tunnel: w145 -> [w606]
    tunnel: w144 -> [w620]
    tunnel: w143 -> [w605]
    tunnel: w142 -> [w619]
    tunnel: w141 -> [w604]
    tunnel: w140 -> [w618]
    tunnel: w139 -> [w603]
    tunnel: w138 -> [w617]
    tunnel: w137 -> [w567]
    tunnel: w136 -> [w616]
    tunnel: w135 -> [w566]
    tunnel: w134 -> [w615]
    tunnel: w133 -> [w565]
    tunnel: w132 -> [w614]
    tunnel: w131 -> [w564]
    tunnel: w130 -> [w613]
    tunnel: w129 -> [w563]
    tunnel: w128 -> [w612]
    tunnel: w127 -> [w562]
    tunnel: w126 -> [w611]
    tunnel: w125 -> [w561]
    tunnel: w124 -> [w625]
    tunnel: w123 -> [w560]
    tunnel: w122 -> [w626]
    stop <- w643 stop-if-true
    w572 = 0.99 ("lower limit")
    w573 = 5.1 ("upper limit")
    w568 = TRUE ("return elements? (F)")
    w706 = TRUE ("y")
    w715 = TRUE ("y")
    w730 = TRUE ("y")
    n287 = local read "Time has Elapsed"() -> (w727:bool)
    n288 = Not And(1:"reset 2", 2:w730) -> (0:w733:bool)
    n289 = Not And(1:w730, 2:w727) -> (0:w728:bool)
    n290 = Build Array("CH1(V)" ("element"), "CH1", "CH2(V)" ("element"), "CH2 2", "CH3(V)" ("element"), "CH3", "CH4(V)" ("element"), "CH4 2", "CH5(V)" ("element"), "CH5", "CH6(V)" ("element"), "CH6", "CH7(V)" ("element"), "CH7", "CH8(V)" ("element"), "CH8", "CH9(V)" ("element"), "CH9", "CH10(V)" ("element"), "CH10", "CH11(V)" ("element"), "CH11", "CH12(V)" ("element"), "CH12", "CH13(V)" ("element"), "CH13", "CH14(V)" ("element"), "CH14", "CH15(V)" ("element"), "CH15", "CH16(V)" ("element"), "CH16") -> (→"appended array":string[])
    n291 = feedback #1() -> (w731:bool)  [unwired: 1 in]
    n292 = Not And(1:w731, 2:w728) -> (0:w734:bool)
    "reset" <- w734
    n293 = Not And(1:w733, 2:w734) -> (0:w732:bool)
    "q'" <- w732
    n294 = feedback-in #1(w732) -> ()
    n295 = case shown="True" "Guardar Configuracion" {
      frame False {
      }
      frame True {
        w1016 = "Offsets" ("section")
        w1015 = TRUE ("use system decimal point (T)")
        w1082 = TRUE ("write raw string? (F)")
        w1049 = "Pendientes" ("section")
        w1085 = "Nombres_Canales" ("section")
        n296 = call <vilib>:"Open Config Data.vi"("create file if necessary (T)"=TRUE, "configuration file path"=path "C:/Users/Zulueta/Documents/Pasantia/Configuracion_16Canales") -> ("error out"=w1184:errorcluster, "refnum"=w1180:T4)  [unwired: 7 in, 1 out]
        n297 = local read "CH1"() -> (w1196:string)
        n298 = call-poly <vilib>:"Write Key.vi"("write raw string? (F)"=w1082, "section"=w1085, "error in (no error)"=w1184, "value"=w1196, "key"="C1", "refnum"=w1180) -> ("error out"=w1185:errorcluster, "refnum out"=w1181:T4)  [unwired: 3 in, 1 out]
        n299 = local read "CH2"() -> (w1197:string)
        n300 = call-poly <vilib>:"Write Key.vi"("write raw string? (F)"=w1082, "section"=w1085, "error in (no error)"=w1185, "value"=w1197, "key"="C2", "refnum"=w1181) -> ("error out"=w1186:errorcluster, "refnum out"=w1182:T4)  [unwired: 3 in, 1 out]
        n301 = local read "CH3"() -> (w1198:string)
        n302 = call-poly <vilib>:"Write Key.vi"("write raw string? (F)"=w1082, "section"=w1085, "error in (no error)"=w1186, "value"=w1198, "key"="C3", "refnum"=w1182) -> ("error out"=w1187:errorcluster, "refnum out"=w1183:T4)  [unwired: 3 in, 1 out]
        n303 = local read "CH4"() -> (w1199:string)
        n304 = call-poly <vilib>:"Write Key.vi"("write raw string? (F)"=w1082, "section"=w1085, "error in (no error)"=w1187, "value"=w1199, "key"="C4", "refnum"=w1183) -> ("error out"=w1188:errorcluster, "refnum out"=w1190:T4)  [unwired: 3 in, 1 out]
        n305 = local read "CH5"() -> (w1200:string)
        n306 = call-poly <vilib>:"Write Key.vi"("write raw string? (F)"=w1082, "section"=w1085, "error in (no error)"=w1188, "value"=w1200, "key"="C5", "refnum"=w1190) -> ("error out"=w1189:errorcluster, "refnum out"=w1191:T4)  [unwired: 3 in, 1 out]
        n307 = local read "CH6"() -> (w1201:string)
        n308 = call-poly <vilib>:"Write Key.vi"("write raw string? (F)"=w1082, "section"=w1085, "error in (no error)"=w1189, "value"=w1201, "key"="C6", "refnum"=w1191) -> ("error out"=w1192:errorcluster, "refnum out"=w1193:T4)  [unwired: 3 in, 1 out]
        n309 = local read "CH7"() -> (w1202:string)
        n310 = call-poly <vilib>:"Write Key.vi"("write raw string? (F)"=w1082, "section"=w1085, "error in (no error)"=w1192, "value"=w1202, "key"="C7", "refnum"=w1193) -> ("error out"=w1195:errorcluster, "refnum out"=w1194:T4)  [unwired: 3 in, 1 out]
        n311 = local read "CH8"() -> (w1118:string)
        n312 = call-poly <vilib>:"Write Key.vi"("write raw string? (F)"=w1082, "section"=w1085, "error in (no error)"=w1195, "value"=w1118, "key"="C8", "refnum"=w1194) -> ("error out"=w1112:errorcluster, "refnum out"=w1113:T4)  [unwired: 3 in, 1 out]
        n313 = local read "CH9"() -> (w1117:string)
        n314 = call-poly <vilib>:"Write Key.vi"("write raw string? (F)"=w1082, "section"=w1085, "error in (no error)"=w1112, "value"=w1117, "key"="C9", "refnum"=w1113) -> ("error out"=w1110:errorcluster, "refnum out"=w1111:T4)  [unwired: 3 in, 1 out]
        n315 = local read "CH10"() -> (w1114:string)
        n316 = call-poly <vilib>:"Write Key.vi"("write raw string? (F)"=w1082, "section"=w1085, "error in (no error)"=w1110, "value"=w1114, "key"="C10", "refnum"=w1111) -> ("error out"=w1108:errorcluster, "refnum out"=w1109:T4)  [unwired: 3 in, 1 out]
        n317 = local read "CH11"() -> (w1106:string)
        n318 = call-poly <vilib>:"Write Key.vi"("write raw string? (F)"=w1082, "section"=w1085, "error in (no error)"=w1108, "value"=w1106, "key"="C11", "refnum"=w1109) -> ("error out"=w1100:errorcluster, "refnum out"=w1101:T4)  [unwired: 3 in, 1 out]
        n319 = local read "CH12"() -> (w1104:string)
        n320 = call-poly <vilib>:"Write Key.vi"("write raw string? (F)"=w1082, "section"=w1085, "error in (no error)"=w1100, "value"=w1104, "key"="C12", "refnum"=w1101) -> ("error out"=w1098:errorcluster, "refnum out"=w1099:T4)  [unwired: 3 in, 1 out]
        n321 = local read "CH13"() -> (w1103:string)
        n322 = call-poly <vilib>:"Write Key.vi"("write raw string? (F)"=w1082, "section"=w1085, "error in (no error)"=w1098, "value"=w1103, "key"="C13", "refnum"=w1099) -> ("error out"=w1097:errorcluster, "refnum out"=w1096:T4)  [unwired: 3 in, 1 out]
        n323 = local read "CH14"() -> (w1095:string)
        n324 = call-poly <vilib>:"Write Key.vi"("write raw string? (F)"=w1082, "section"=w1085, "error in (no error)"=w1097, "value"=w1095, "key"="C14", "refnum"=w1096) -> ("error out"=w1091:errorcluster, "refnum out"=w1090:T4)  [unwired: 3 in, 1 out]
        n325 = local read "CH15"() -> (w1093:string)
        n326 = call-poly <vilib>:"Write Key.vi"("write raw string? (F)"=w1082, "section"=w1085, "error in (no error)"=w1091, "value"=w1093, "key"="C15", "refnum"=w1090) -> ("error out"=w1088:errorcluster, "refnum out"=w1089:T4)  [unwired: 3 in, 1 out]
        n327 = local read "CH16"() -> (w1087:string)
        n328 = call-poly <vilib>:"Write Key.vi"("write raw string? (F)"=w1082, "section"=w1085, "error in (no error)"=w1088, "value"=w1087, "key"="C16", "refnum"=w1089) -> ("error out"=w1083:errorcluster, "refnum out"=w1084:T4)  [unwired: 3 in, 1 out]
        n329 = local read "m1"() -> (w1171:dbl)
        n330 = call-poly <vilib>:"Write Key.vi"("use system decimal point (T)"=w1015, "section"=w1049, "error in (no error)"=w1083, "value"=w1171, "key"="M1", "refnum"=w1084) -> ("error out"=w1177:errorcluster, "refnum out"=w1178:T4)  [unwired: 3 in, 1 out]
        n331 = local read "m2"() -> (w1170:dbl)
        n332 = call-poly <vilib>:"Write Key.vi"("use system decimal point (T)"=w1015, "section"=w1049, "error in (no error)"=w1177, "value"=w1170, "key"="M2", "refnum"=w1178) -> ("error out"=w1175:errorcluster, "refnum out"=w1176:T4)  [unwired: 3 in, 1 out]
        n333 = local read "m3"() -> (w1168:dbl)
        n334 = call-poly <vilib>:"Write Key.vi"("use system decimal point (T)"=w1015, "section"=w1049, "error in (no error)"=w1175, "value"=w1168, "key"="M3", "refnum"=w1176) -> ("error out"=w1173:errorcluster, "refnum out"=w1174:T4)  [unwired: 3 in, 1 out]
        n335 = local read "m4"() -> (w1166:dbl)
        n336 = call-poly <vilib>:"Write Key.vi"("use system decimal point (T)"=w1015, "section"=w1049, "error in (no error)"=w1173, "value"=w1166, "key"="M4", "refnum"=w1174) -> ("error out"=w1163:errorcluster, "refnum out"=w1164:T4)  [unwired: 3 in, 1 out]
        n337 = local read "m5"() -> (w1162:dbl)
        n338 = call-poly <vilib>:"Write Key.vi"("use system decimal point (T)"=w1015, "section"=w1049, "error in (no error)"=w1163, "value"=w1162, "key"="M5", "refnum"=w1164) -> ("error out"=w1157:errorcluster, "refnum out"=w1158:T4)  [unwired: 3 in, 1 out]
        n339 = local read "m6"() -> (w1160:dbl)
        n340 = call-poly <vilib>:"Write Key.vi"("use system decimal point (T)"=w1015, "section"=w1049, "error in (no error)"=w1157, "value"=w1160, "key"="M6", "refnum"=w1158) -> ("error out"=w1155:errorcluster, "refnum out"=w1156:T4)  [unwired: 3 in, 1 out]
        n341 = local read "m7"() -> (w1154:dbl)
        n342 = call-poly <vilib>:"Write Key.vi"("use system decimal point (T)"=w1015, "section"=w1049, "error in (no error)"=w1155, "value"=w1154, "key"="M7", "refnum"=w1156) -> ("error out"=w1151:errorcluster, "refnum out"=w1152:T4)  [unwired: 3 in, 1 out]
        n343 = local read "m8"() -> (w1150:dbl)
        n344 = call-poly <vilib>:"Write Key.vi"("use system decimal point (T)"=w1015, "section"=w1049, "error in (no error)"=w1151, "value"=w1150, "key"="M8", "refnum"=w1152) -> ("error out"=w1078:errorcluster, "refnum out"=w1079:T4)  [unwired: 3 in, 1 out]
        n345 = local read "m9"() -> (w1081:dbl)
        n346 = call-poly <vilib>:"Write Key.vi"("use system decimal point (T)"=w1015, "section"=w1049, "error in (no error)"=w1078, "value"=w1081, "key"="M9", "refnum"=w1079) -> ("error out"=w1070:errorcluster, "refnum out"=w1071:T4)  [unwired: 3 in, 1 out]
        n347 = local read "m10"() -> (w1077:dbl)
        n348 = call-poly <vilib>:"Write Key.vi"("use system decimal point (T)"=w1015, "section"=w1049, "error in (no error)"=w1070, "value"=w1077, "key"="M10", "refnum"=w1071) -> ("error out"=w1069:errorcluster, "refnum out"=w1072:T4)  [unwired: 3 in, 1 out]
        n349 = local read "m11"() -> (w1075:dbl)
        n350 = call-poly <vilib>:"Write Key.vi"("use system decimal point (T)"=w1015, "section"=w1049, "error in (no error)"=w1069, "value"=w1075, "key"="M11", "refnum"=w1072) -> ("error out"=w1068:errorcluster, "refnum out"=w1073:T4)  [unwired: 3 in, 1 out]
        n351 = local read "m12"() -> (w1067:dbl)
        n352 = call-poly <vilib>:"Write Key.vi"("use system decimal point (T)"=w1015, "section"=w1049, "error in (no error)"=w1068, "value"=w1067, "key"="M12", "refnum"=w1073) -> ("error out"=w1059:errorcluster, "refnum out"=w1058:T4)  [unwired: 3 in, 1 out]
        n353 = local read "m13"() -> (w1064:dbl)
        n354 = call-poly <vilib>:"Write Key.vi"("use system decimal point (T)"=w1015, "section"=w1049, "error in (no error)"=w1059, "value"=w1064, "key"="M13", "refnum"=w1058) -> ("error out"=w1056:errorcluster, "refnum out"=w1057:T4)  [unwired: 3 in, 1 out]
        n355 = local read "m14"() -> (w1062:dbl)
        n356 = call-poly <vilib>:"Write Key.vi"("use system decimal point (T)"=w1015, "section"=w1049, "error in (no error)"=w1056, "value"=w1062, "key"="M14", "refnum"=w1057) -> ("error out"=w1055:errorcluster, "refnum out"=w1054:T4)  [unwired: 3 in, 1 out]
        n357 = local read "m15"() -> (w1060:dbl)
        n358 = call-poly <vilib>:"Write Key.vi"("use system decimal point (T)"=w1015, "section"=w1049, "error in (no error)"=w1055, "value"=w1060, "key"="M15", "refnum"=w1054) -> ("error out"=w1050:errorcluster, "refnum out"=w1051:T4)  [unwired: 3 in, 1 out]
        n359 = local read "m16"() -> (w1052:dbl)
        n360 = call-poly <vilib>:"Write Key.vi"("use system decimal point (T)"=w1015, "section"=w1049, "error in (no error)"=w1050, "value"=w1052, "key"="M16", "refnum"=w1051) -> ("error out"=w1047:errorcluster, "refnum out"=w1048:T4)  [unwired: 3 in, 1 out]
        n361 = local read "b1"() -> (w1147:dbl)
        n362 = call-poly <vilib>:"Write Key.vi"("use system decimal point (T)"=w1015, "section"=w1016, "error in (no error)"=w1047, "value"=w1147, "key"="B1", "refnum"=w1048) -> ("error out"=w1145:errorcluster, "refnum out"=w1146:T4)  [unwired: 3 in, 1 out]
        n363 = local read "b2"() -> (w1143:dbl)
        n364 = call-poly <vilib>:"Write Key.vi"("use system decimal point (T)"=w1015, "section"=w1016, "error in (no error)"=w1145, "value"=w1143, "key"="B2", "refnum"=w1146) -> ("error out"=w1140:errorcluster, "refnum out"=w1141:T4)  [unwired: 3 in, 1 out]
        n365 = local read "b3"() -> (w1142:dbl)
        n366 = call-poly <vilib>:"Write Key.vi"("use system decimal point (T)"=w1015, "section"=w1016, "error in (no error)"=w1140, "value"=w1142, "key"="B3", "refnum"=w1141) -> ("error out"=w1137:errorcluster, "refnum out"=w1138:T4)  [unwired: 3 in, 1 out]
        n367 = local read "b4"() -> (w1136:dbl)
        n368 = call-poly <vilib>:"Write Key.vi"("use system decimal point (T)"=w1015, "section"=w1016, "error in (no error)"=w1137, "value"=w1136, "key"="B4", "refnum"=w1138) -> ("error out"=w1134:errorcluster, "refnum out"=w1133:T4)  [unwired: 3 in, 1 out]
        n369 = local read "b5"() -> (w1132:dbl)
        n370 = call-poly <vilib>:"Write Key.vi"("use system decimal point (T)"=w1015, "section"=w1016, "error in (no error)"=w1134, "value"=w1132, "key"="B5", "refnum"=w1133) -> ("error out"=w1130:errorcluster, "refnum out"=w1129:T4)  [unwired: 3 in, 1 out]
        n371 = local read "b6"() -> (w1128:dbl)
        n372 = call-poly <vilib>:"Write Key.vi"("use system decimal point (T)"=w1015, "section"=w1016, "error in (no error)"=w1130, "value"=w1128, "key"="B6", "refnum"=w1129) -> ("error out"=w1125:errorcluster, "refnum out"=w1126:T4)  [unwired: 3 in, 1 out]
        n373 = local read "b7"() -> (w1124:dbl)
        n374 = call-poly <vilib>:"Write Key.vi"("use system decimal point (T)"=w1015, "section"=w1016, "error in (no error)"=w1125, "value"=w1124, "key"="B7", "refnum"=w1126) -> ("error out"=w1121:errorcluster, "refnum out"=w1122:T4)  [unwired: 3 in, 1 out]
        n375 = local read "b8"() -> (w1120:dbl)
        n376 = call-poly <vilib>:"Write Key.vi"("use system decimal point (T)"=w1015, "section"=w1016, "error in (no error)"=w1121, "value"=w1120, "key"="B8", "refnum"=w1122) -> ("error out"=w1045:errorcluster, "refnum out"=w1046:T4)  [unwired: 3 in, 1 out]
        n377 = local read "b9"() -> (w1044:dbl)
        n378 = call-poly <vilib>:"Write Key.vi"("use system decimal point (T)"=w1015, "section"=w1016, "error in (no error)"=w1045, "value"=w1044, "key"="B9", "refnum"=w1046) -> ("error out"=w1042:errorcluster, "refnum out"=w1041:T4)  [unwired: 3 in, 1 out]
        n379 = local read "b10"() -> (w1039:dbl)
        n380 = call-poly <vilib>:"Write Key.vi"("use system decimal point (T)"=w1015, "section"=w1016, "error in (no error)"=w1042, "value"=w1039, "key"="B10", "refnum"=w1041) -> ("error out"=w1037:errorcluster, "refnum out"=w1038:T4)  [unwired: 3 in, 1 out]
        n381 = local read "b11"() -> (w1035:dbl)
        n382 = call-poly <vilib>:"Write Key.vi"("use system decimal point (T)"=w1015, "section"=w1016, "error in (no error)"=w1037, "value"=w1035, "key"="B11", "refnum"=w1038) -> ("error out"=w1031:errorcluster, "refnum out"=w1032:T4)  [unwired: 3 in, 1 out]
        n383 = local read "b12"() -> (w1034:dbl)
        n384 = call-poly <vilib>:"Write Key.vi"("use system decimal point (T)"=w1015, "section"=w1016, "error in (no error)"=w1031, "value"=w1034, "key"="B12", "refnum"=w1032) -> ("error out"=w1028:errorcluster, "refnum out"=w1027:T4)  [unwired: 3 in, 1 out]
        n385 = local read "b13"() -> (w1029:dbl)
        n386 = call-poly <vilib>:"Write Key.vi"("use system decimal point (T)"=w1015, "section"=w1016, "error in (no error)"=w1028, "value"=w1029, "key"="B13", "refnum"=w1027) -> ("error out"=w1023:errorcluster, "refnum out"=w1024:T4)  [unwired: 3 in, 1 out]
        n387 = local read "b14"() -> (w1026:dbl)
        n388 = call-poly <vilib>:"Write Key.vi"("use system decimal point (T)"=w1015, "section"=w1016, "error in (no error)"=w1023, "value"=w1026, "key"="B14", "refnum"=w1024) -> ("error out"=w1022:errorcluster, "refnum out"=w1021:T4)  [unwired: 3 in, 1 out]
        n389 = local read "b15"() -> (w1019:dbl)
        n390 = call-poly <vilib>:"Write Key.vi"("use system decimal point (T)"=w1015, "section"=w1016, "error in (no error)"=w1022, "value"=w1019, "key"="B15", "refnum"=w1021) -> ("error out"=w1013:errorcluster, "refnum out"=w1014:T4)  [unwired: 3 in, 1 out]
        n391 = local read "b16"() -> (w1018:dbl)
        n392 = call-poly <vilib>:"Write Key.vi"("use system decimal point (T)"=w1015, "section"=w1016, "error in (no error)"=w1013, "value"=w1018, "key"="B16", "refnum"=w1014) -> ("error out"=w1012:errorcluster, "refnum out"=w1011:T4)  [unwired: 3 in, 1 out]
        n393 = call <vilib>:"Close Config Data.vi"("error in (no error)"=w1012, "refnum"=w1011) -> ()  [unwired: 8 in, 2 out]
      }
    }
    n394 = local read "Time has Elapsed 2"() -> (w711:bool)
    n395 = Not And(1:"?", 2:w715) -> (0:w718:bool)
    n396 = Not And(1:w715, 2:w711) -> (0:w714:bool)
    n397 = feedback #2() -> (w716:bool)  [unwired: 1 in]
    n398 = Not And(1:w716, 2:w714) -> (0:w713:bool)
    "reset2" <- w713
    n399 = Not And(1:w718, 2:w713) -> (0:w717:bool)
    "q2'" <- w717
    n400 = feedback-in #2(w717) -> ()
    n401 = Get Queue Status(queue=w609, return elements? (F)=w568) -> (elements=w650:dbl[])  [unwired: 1 in, 7 out]
    n402 = Get Queue Status(queue=w608, return elements? (F)=w568) -> (elements=w649:dbl[])  [unwired: 1 in, 7 out]
    n403 = Get Queue Status(queue=w607, return elements? (F)=w568) -> (elements=w648:dbl[])  [unwired: 1 in, 7 out]
    n404 = Get Queue Status(queue=w610, return elements? (F)=w568) -> (# elements in queue=w693:i32, elements=w651:dbl[])  [unwired: 1 in, 6 out]
    n405 = Get Queue Status(queue=w606, return elements? (F)=w568) -> (elements=w647:dbl[])  [unwired: 1 in, 7 out]
    n406 = Get Queue Status(queue=w605, return elements? (F)=w568) -> (elements=w645:dbl[])  [unwired: 1 in, 7 out]
    n407 = Get Queue Status(queue=w604, return elements? (F)=w568) -> (elements=w646:dbl[])  [unwired: 1 in, 7 out]
    n408 = Get Queue Status(queue=w603, return elements? (F)=w568) -> (elements=w644:dbl[])  [unwired: 1 in, 7 out]
    n409 = Get Queue Status(queue=w567, return elements? (F)=w568) -> (elements=w602:dbl[])  [unwired: 1 in, 7 out]
    n410 = Get Queue Status(queue=w566, return elements? (F)=w568) -> (elements=w601:dbl[])  [unwired: 1 in, 7 out]
    n411 = Get Queue Status(queue=w565, return elements? (F)=w568) -> (elements=w600:dbl[])  [unwired: 1 in, 7 out]
    n412 = Get Queue Status(queue=w564, return elements? (F)=w568) -> (elements=w599:dbl[])  [unwired: 1 in, 7 out]
    n413 = Get Queue Status(queue=w563, return elements? (F)=w568) -> (elements=w598:dbl[])  [unwired: 1 in, 7 out]
    n414 = Get Queue Status(queue=w562, return elements? (F)=w568) -> (elements=w597:dbl[])  [unwired: 1 in, 7 out]
    n415 = Get Queue Status(queue=w561, return elements? (F)=w568) -> (elements=w596:dbl[])  [unwired: 1 in, 7 out]
    n416 = Get Queue Status(queue=w560, return elements? (F)=w568) -> (elements=w575:dbl[])  [unwired: 1 in, 7 out]
    n417 = property on="index" class="DigNum (strict)"("Value"=w693) -> ()  [unwired: 2 in, 2 out]
    n418 = local read "Iniciar"() -> (w704:bool)
    n419 = Index Array(array=w651, index="index") -> (element=w675:dbl)
    n420 = Index Array(array=w650, index="index") -> (element=w674:dbl)
    n421 = Index Array(array=w649, index="index") -> (element=w673:dbl)
    n422 = Index Array(array=w648, index="index") -> (element=w672:dbl)
    n423 = Index Array(array=w647, index="index") -> (element=w671:dbl)
    n424 = Index Array(array=w645, index="index") -> (element=w670:dbl)
    n425 = Index Array(array=w646, index="index") -> (element=w669:dbl)
    n426 = Index Array(array=w644, index="index") -> (element=w668:dbl)
    n427 = Index Array(array=w602) -> (element=w595:dbl)  [unwired: 1 in]
    n428 = Index Array(array=w601) -> (element=w594:dbl)  [unwired: 1 in]
    n429 = Index Array(array=w600) -> (element=w593:dbl)  [unwired: 1 in]
    n430 = Index Array(array=w599) -> (element=w592:dbl)  [unwired: 1 in]
    n431 = Index Array(array=w598) -> (element=w591:dbl)  [unwired: 1 in]
    n432 = Index Array(array=w597) -> (element=w590:dbl)  [unwired: 1 in]
    n433 = Index Array(array=w596) -> (element=w589:dbl)  [unwired: 1 in]
    n434 = Index Array(array=w575) -> (element=w574:dbl)  [unwired: 1 in]
    n435 = Not(x=w704) -> (.not. x?=w703:bool)
    n436 = In Range and Coerce(upper limit=w573, x=w675, lower limit=w572) -> (In Range?=w667:bool)  [unwired: 1 out]
    n437 = In Range and Coerce(upper limit=w573, x=w674, lower limit=w572) -> (In Range?=w666:bool)  [unwired: 1 out]
    n438 = In Range and Coerce(upper limit=w573, x=w673, lower limit=w572) -> (In Range?=w665:bool)  [unwired: 1 out]
    n439 = In Range and Coerce(upper limit=w573, x=w672, lower limit=w572) -> (In Range?=w664:bool)  [unwired: 1 out]
    n440 = In Range and Coerce(upper limit=w573, x=w671, lower limit=w572) -> (In Range?=w663:bool)  [unwired: 1 out]
    n441 = In Range and Coerce(upper limit=w573, x=w670, lower limit=w572) -> (In Range?=w662:bool)  [unwired: 1 out]
    n442 = In Range and Coerce(upper limit=w573, x=w669, lower limit=w572) -> (In Range?=w661:bool)  [unwired: 1 out]
    n443 = In Range and Coerce(upper limit=w573, x=w668, lower limit=w572) -> (In Range?=w660:bool)  [unwired: 1 out]
    n444 = In Range and Coerce(upper limit=w573, x=w595, lower limit=w572) -> (In Range?=w588:bool)  [unwired: 1 out]
    n445 = In Range and Coerce(upper limit=w573, x=w594, lower limit=w572) -> (In Range?=w587:bool)  [unwired: 1 out]
    n446 = In Range and Coerce(upper limit=w573, x=w593, lower limit=w572) -> (In Range?=w586:bool)  [unwired: 1 out]
    n447 = In Range and Coerce(upper limit=w573, x=w592, lower limit=w572) -> (In Range?=w585:bool)  [unwired: 1 out]
    n448 = In Range and Coerce(upper limit=w573, x=w591, lower limit=w572) -> (In Range?=w584:bool)  [unwired: 1 out]
    n449 = In Range and Coerce(upper limit=w573, x=w590, lower limit=w572) -> (In Range?=w583:bool)  [unwired: 1 out]
    n450 = In Range and Coerce(upper limit=w573, x=w589, lower limit=w572) -> (In Range?=w582:bool)  [unwired: 1 out]
    n451 = In Range and Coerce(upper limit=w573, x=w574, lower limit=w572) -> (In Range?=w571:bool)  [unwired: 1 out]
    n452 = Not And(1:w704, 2:w706) -> (0:w710:bool)
    n453 = Not And(1:w706, 2:w703) -> (0:w707:bool)
    n454 = Not(x=w667) -> (.not. x?=w659:bool)
    n455 = Not(x=w666) -> (.not. x?=w658:bool)
    n456 = Not(x=w665) -> (.not. x?=w657:bool)
    n457 = Not(x=w664) -> (.not. x?=w656:bool)
    n458 = Not(x=w663) -> (.not. x?=w655:bool)
    n459 = Not(x=w662) -> (.not. x?=w654:bool)
    n460 = Not(x=w661) -> (.not. x?=w653:bool)
    n461 = Not(x=w660) -> (.not. x?=w652:bool)
    n462 = Not(x=w588) -> (.not. x?=w581:bool)
    n463 = Not(x=w587) -> (.not. x?=w580:bool)
    n464 = Not(x=w586) -> (.not. x?=w579:bool)
    n465 = Not(x=w585) -> (.not. x?=w578:bool)
    n466 = Not(x=w584) -> (.not. x?=w577:bool)
    n467 = Not(x=w583) -> (.not. x?=w576:bool)
    n468 = Not(x=w582) -> (.not. x?=w570:bool)
    n469 = Not(x=w571) -> (.not. x?=w569:bool)
    n470 = feedback #3() -> (w708:bool)  [unwired: 1 in]
    n471 = Not And(1:w708, 2:w707) -> (0:w705:bool)
    "reset3" <- w705
    n472 = Not And(1:w710, 2:w705) -> (0:w709:bool)
    n473 = feedback-in #3(w709) -> ()
    n474 = Build Array(w659, w658, w657, w656, w655, w654, w653, w652, w581, w580, w579, w578, w577, w576, w570, w569) -> (w559:bool[])
    n475 = local read "q'"() -> (w678:bool)
    n476 = local read "reset3"() -> (w690:bool)
    n477 = local read "q2'"() -> (w677:bool)
    n478 = call "DAQ Assistant2"("data"=w559) -> ()  [unwired: 17 in, 2 out]
    n479 = case shown="True" w678 {
      frame False {
      }
      frame True {
        w1218 = TRUE ("s")
        n480 = local read "reset"() -> (w1221:bool)
        n481 = local read "Time"() -> (w1223:dbl)
        n482 = call "Elapsed Time"("Time Target (s)"=w1223, "Reset"=w1221) -> ("Elapsed Time (s)"=w1220:dbl, "Time has Elapsed"=→"Time has Elapsed":bool)  [unwired: 10 in, 6 out]
        "Tiempo" <- w1220
        n483 = property on="Tiempo" class="DigNum (strict)"("Value"=w1220) -> ()  [unwired: 2 in, 2 out]
        n484 = property on="Datapath" class="Bool (strict)"("Value"=w1218) -> ()  [unwired: 2 in, 2 out]
        n485 = property on="Path1" class="Bool (strict)"("Value"=FALSE ("Boolean 19")) -> ()  [unwired: 2 in, 2 out]
        n486 = property on="Guardar" class="Bool (strict)"("Value"=w1218) -> ()  [unwired: 2 in, 2 out]
        n487 = property on="Path2" class="Bool (strict)"("Value"=w1218) -> ()  [unwired: 2 in, 2 out]
      }
    }
    n488 = case shown="True" "Iniciar" {
      tunnel: w690 -> [_ w1226]
      frame False {
      }
      frame True {
        w1224 = TRUE ("s")
        n489 = call "Elapsed Time3"("Reset"=w1226) -> ("Elapsed Time (s)"=w1225:dbl)  [unwired: 11 in, 7 out]
        "Tiempo" <- w1225
        n490 = property on="Tiempo" class="DigNum (strict)"("Value"=w1225) -> ()  [unwired: 2 in, 2 out]
        n491 = property on="Datapath" class="Bool (strict)"("Value"=w1224) -> ()  [unwired: 2 in, 2 out]
        n492 = property on="Path1" class="Bool (strict)"("Value"=w1224) -> ()  [unwired: 2 in, 2 out]
        n493 = property on="Guardar" class="Bool (strict)"("Value"=w1224) -> ()  [unwired: 2 in, 2 out]
        n494 = property on="Path2" class="Bool (strict)"("Value"=w1224) -> ()  [unwired: 2 in, 2 out]
      }
    }
    n495 = case shown="True" w677 {
      frame False {
      }
      frame True {
        w1213 = FALSE ("s")
        n496 = local read "reset2"() -> (w1215:bool)
        n497 = local read "Time"() -> (w1217:dbl)
        n498 = call "Elapsed Time2"("Time Target (s)"=w1217, "Reset"=w1215) -> ("Elapsed Time (s)"=w1212:dbl, "Time has Elapsed"=→"Time has Elapsed 2":bool)  [unwired: 10 in, 6 out]
        "Tiempo" <- w1212
        n499 = property on="Tiempo" class="DigNum (strict)"("Value"=w1212) -> ()  [unwired: 2 in, 2 out]
        n500 = property on="Datapath" class="Bool (strict)"("Value"=w1213) -> ()  [unwired: 2 in, 2 out]
        n501 = property on="Path2" class="Bool (strict)"("Value"=w1213) -> ()  [unwired: 2 in, 2 out]
        n502 = property on="Guardar" class="Bool (strict)"("Value"=TRUE ("y")) -> ()  [unwired: 2 in, 2 out]
      }
    }
    n503 = case shown="\"Minutos\"" "Tiempo \nde adquisición" {
      tunnel: [w1229 w1232 w1239] -> w736
      frame "Segundos", Default {
        n504 = Equal To 0?(x="?") -> (x = 0?=w1228:bool)
        n505 = case shown="True" w1228 {
          tunnel: [w1230 -1] -> w1229
          tunnel: "?" -> [w1230 _]
          frame False {
          }
          frame True {
          }
        }
      }
      frame "Minutos" {
        n506 = Equal To 0?(x="?") -> (x = 0?=w1234:bool)
        n507 = case shown="False" w1234 {
          tunnel: [w1235 -1] -> w1232
          tunnel: "?" -> [w1237 _]
          frame False {
            n508 = Multiply(x=w1237, y=60.0) -> (x*y=w1235:dbl)
          }
          frame True {
          }
        }
      }
      frame "Horas" {
        n509 = Equal To 0?(x="?") -> (x = 0?=w1241:bool)
        n510 = case shown="False" w1241 {
          tunnel: [w1242 -1] -> w1239
          tunnel: "?" -> [w1244 _]
          frame False {
            n511 = Multiply(x=w1244, y=3600.0) -> (x*y=w1242:dbl)
          }
          frame True {
          }
        }
      }
    }
    "Time" <- w736
    n512 = Or(x=w678, y=w677) -> (x .or. y?=w679:bool)
    n513 = Or(x="Iniciar", y=w679) -> (x .or. y?=w687:bool)
    n514 = case shown="False" w687 {
      frame False {
        n515 = property on="index" class="DigNum (strict)"() -> ("Value"=w738:i32)  [unwired: 2 in, 2 out]
        n516 = property on="index 3" class="DigNum (strict)"("Value"=w738) -> ()  [unwired: 2 in, 2 out]
      }
      frame True {
      }
    }
    n517 = Not(x=w687) -> (.not. x?=w692:bool)
    n518 = And(x=w692, y="Guardar") -> (x .and. y?=w691:bool)
    n519 = Select(t=w686, s="Path1", f=w685) -> (s? t:f=w683:refnum<k34>)
    n520 = Select(t=w683, s="Path2", f=w676) -> (s? t:f=w682:refnum<k34>)
    n521 = case shown="True" w691 {
      tunnel: w682 -> [_ w989]
      tunnel: w626 -> [_ w900]
      tunnel: w560 -> [_ w901]
      tunnel: w625 -> [_ w902]
      tunnel: w610 -> [_ w950]
      tunnel: w624 -> [_ w949]
      tunnel: w609 -> [_ w948]
      tunnel: w623 -> [_ w947]
      tunnel: w608 -> [_ w946]
      tunnel: w622 -> [_ w945]
      tunnel: w607 -> [_ w944]
      tunnel: w621 -> [_ w943]
      tunnel: w606 -> [_ w942]
      tunnel: w620 -> [_ w941]
      tunnel: w605 -> [_ w940]
      tunnel: w619 -> [_ w939]
      tunnel: w604 -> [_ w938]
      tunnel: w618 -> [_ w937]
      tunnel: w603 -> [_ w936]
      tunnel: w617 -> [_ w935]
      tunnel: w567 -> [_ w923]
      tunnel: w616 -> [_ w922]
      tunnel: w566 -> [_ w921]
      tunnel: w615 -> [_ w920]
      tunnel: w565 -> [_ w919]
      tunnel: w614 -> [_ w918]
      tunnel: w564 -> [_ w917]
      tunnel: w613 -> [_ w916]
      tunnel: w563 -> [_ w915]
      tunnel: w612 -> [_ w914]
      tunnel: w562 -> [_ w913]
      tunnel: w611 -> [_ w904]
      tunnel: w561 -> [_ w903]
      frame False {
      }
      frame True {
        w835 = enum16{"Sample", "Population"}."Population" ("Weighting (Sample)")
        w905 = TRUE ("return elements? (F)")
        n522 = property on="Tasa de Adquisicion" class="DigNum (strict)"() -> ("Value"=w1009:dbl)  [unwired: 2 in, 2 out]
        n523 = Multiply(x="Tiempo", y=w1009) -> (x*y=w1008:dbl)
        n524 = Round Toward -Infinity(1:w1008) -> (0:w906:dbl)
        n525 = Get Queue Status(queue=w950, return elements? (F)=w905) -> (elements=w1010:dbl[])  [unwired: 1 in, 7 out]
        n526 = Get Queue Status(queue=w949, return elements? (F)=w905) -> (elements=w1007:dbl[])  [unwired: 1 in, 7 out]
        n527 = Get Queue Status(queue=w948, return elements? (F)=w905) -> (elements=w1006:dbl[])  [unwired: 1 in, 7 out]
        n528 = Get Queue Status(queue=w947, return elements? (F)=w905) -> (elements=w1005:dbl[])  [unwired: 1 in, 7 out]
        n529 = Get Queue Status(queue=w946, return elements? (F)=w905) -> (elements=w1004:dbl[])  [unwired: 1 in, 7 out]
        n530 = Get Queue Status(queue=w944, return elements? (F)=w905) -> (elements=w1002:dbl[])  [unwired: 1 in, 7 out]
        n531 = Get Queue Status(queue=w943, return elements? (F)=w905) -> (elements=w1001:dbl[])  [unwired: 1 in, 7 out]
        n532 = Get Queue Status(queue=w942, return elements? (F)=w905) -> (elements=w1000:dbl[])  [unwired: 1 in, 7 out]
        n533 = Get Queue Status(queue=w941, return elements? (F)=w905) -> (elements=w999:dbl[])  [unwired: 1 in, 7 out]
        n534 = Get Queue Status(queue=w940, return elements? (F)=w905) -> (elements=w998:dbl[])  [unwired: 1 in, 7 out]
        n535 = Get Queue Status(queue=w939, return elements? (F)=w905) -> (elements=w997:dbl[])  [unwired: 1 in, 7 out]
        n536 = Get Queue Status(queue=w938, return elements? (F)=w905) -> (elements=w996:dbl[])  [unwired: 1 in, 7 out]
        n537 = Get Queue Status(queue=w937, return elements? (F)=w905) -> (elements=w995:dbl[])  [unwired: 1 in, 7 out]
        n538 = Get Queue Status(queue=w936, return elements? (F)=w905) -> (elements=w994:dbl[])  [unwired: 1 in, 7 out]
        n539 = Get Queue Status(queue=w935, return elements? (F)=w905) -> (elements=w993:dbl[])  [unwired: 1 in, 7 out]
        n540 = Get Queue Status(queue=w923, return elements? (F)=w905) -> (elements=w934:dbl[])  [unwired: 1 in, 7 out]
        n541 = Get Queue Status(queue=w922, return elements? (F)=w905) -> (elements=w933:dbl[])  [unwired: 1 in, 7 out]
        n542 = Get Queue Status(queue=w921, return elements? (F)=w905) -> (elements=w932:dbl[])  [unwired: 1 in, 7 out]
        n543 = Get Queue Status(queue=w920, return elements? (F)=w905) -> (elements=w931:dbl[])  [unwired: 1 in, 7 out]
        n544 = Get Queue Status(queue=w919, return elements? (F)=w905) -> (elements=w930:dbl[])  [unwired: 1 in, 7 out]
        n545 = Get Queue Status(queue=w918, return elements? (F)=w905) -> (elements=w929:dbl[])  [unwired: 1 in, 7 out]
        n546 = Get Queue Status(queue=w917, return elements? (F)=w905) -> (elements=w928:dbl[])  [unwired: 1 in, 7 out]
        n547 = Get Queue Status(queue=w916, return elements? (F)=w905) -> (elements=w927:dbl[])  [unwired: 1 in, 7 out]
        n548 = Get Queue Status(queue=w915, return elements? (F)=w905) -> (elements=w926:dbl[])  [unwired: 1 in, 7 out]
        n549 = Get Queue Status(queue=w914, return elements? (F)=w905) -> (elements=w925:dbl[])  [unwired: 1 in, 7 out]
        n550 = Get Queue Status(queue=w913, return elements? (F)=w905) -> (elements=w924:dbl[])  [unwired: 1 in, 7 out]
        n551 = Get Queue Status(queue=w904, return elements? (F)=w905) -> (elements=w912:dbl[])  [unwired: 1 in, 7 out]
        n552 = Get Queue Status(queue=w903, return elements? (F)=w905) -> (elements=w911:dbl[])  [unwired: 1 in, 7 out]
        n553 = Get Queue Status(queue=w902, return elements? (F)=w905) -> (elements=w910:dbl[])  [unwired: 1 in, 7 out]
        n554 = Get Queue Status(queue=w901, return elements? (F)=w905) -> (elements=w909:dbl[])  [unwired: 1 in, 7 out]
        n555 = Get Queue Status(queue=w900, return elements? (F)=w905) -> (elements=w908:dbl[])  [unwired: 1 in, 7 out]
        n556 = Get Queue Status(queue=w945, return elements? (F)=w905) -> (elements=w1003:dbl[])  [unwired: 1 in, 7 out]
        n557 = Array Subset(array=w1010, index="index 3", length=w906) -> (w834:dbl[])
        n558 = Array Subset(array=w1007, index="index 3", length=w906) -> (w833:dbl[])
        n559 = Array Subset(array=w1006, index="index 3", length=w906) -> (w832:dbl[])
        n560 = Array Subset(array=w1005, index="index 3", length=w906) -> (w831:dbl[])
        n561 = Array Subset(array=w1004, index="index 3", length=w906) -> (w830:dbl[])
        n562 = Array Subset(array=w1003, index="index 3", length=w906) -> (w829:dbl[])
        n563 = Array Subset(array=w1002, index="index 3", length=w906) -> (w828:dbl[])
        n564 = Array Subset(array=w1001, index="index 3", length=w906) -> (w827:dbl[])
        n565 = Array Subset(array=w1000, index="index 3", length=w906) -> (w826:dbl[])
        n566 = Array Subset(array=w999, index="index 3", length=w906) -> (w825:dbl[])
        n567 = Array Subset(array=w998, index="index 3", length=w906) -> (w824:dbl[])
        n568 = Array Subset(array=w997, index="index 3", length=w906) -> (w823:dbl[])
        n569 = Array Subset(array=w996, index="index 3", length=w906) -> (w822:dbl[])
        n570 = Array Subset(array=w995, index="index 3", length=w906) -> (w821:dbl[])
        n571 = Array Subset(array=w994, index="index 3", length=w906) -> (w820:dbl[])
        n572 = Array Subset(array=w993, index="index 3", length=w906) -> (w819:dbl[])
        n573 = Array Subset(array=w934, index="index 3", length=w906) -> (w818:dbl[])
        n574 = Array Subset(array=w933, index="index 3", length=w906) -> (w817:dbl[])
        n575 = Array Subset(array=w932, index="index 3", length=w906) -> (w816:dbl[])
        n576 = Array Subset(array=w931, index="index 3", length=w906) -> (w815:dbl[])
        n577 = Array Subset(array=w930, index="index 3", length=w906) -> (w814:dbl[])
        n578 = Array Subset(array=w929, index="index 3", length=w906) -> (w813:dbl[])
        n579 = Array Subset(array=w928, index="index 3", length=w906) -> (w812:dbl[])
        n580 = Array Subset(array=w927, index="index 3", length=w906) -> (w811:dbl[])
        n581 = Array Subset(array=w926, index="index 3", length=w906) -> (w810:dbl[])
        n582 = Array Subset(array=w925, index="index 3", length=w906) -> (w809:dbl[])
        n583 = Array Subset(array=w924, index="index 3", length=w906) -> (w808:dbl[])
        n584 = Array Subset(array=w912, index="index 3", length=w906) -> (w807:dbl[])
        n585 = Array Subset(array=w911, index="index 3", length=w906) -> (w806:dbl[])
        n586 = Array Subset(array=w910, index="index 3", length=w906) -> (w805:dbl[])
        n587 = Array Subset(array=w909, index="index 3", length=w906) -> (w804:dbl[])
        n588 = Array Subset(array=w908, index="index 3", length=w906) -> (w803:dbl[])
        n589 = call "Convert to Dynamic Data"("Array"=w834) -> ("Dynamic Data Type"=w899:dynamicdata)  [unwired: 3 in]
        n590 = call "Convert to Dynamic Data2"("Array"=w833) -> ("Dynamic Data Type"=w898:dynamicdata)  [unwired: 3 in]
        n591 = call "Convert to Dynamic Data3"("Array"=w832) -> ("Dynamic Data Type"=w897:dynamicdata)  [unwired: 3 in]
        n592 = call "Convert to Dynamic Data4"("Array"=w831) -> ("Dynamic Data Type"=w896:dynamicdata)  [unwired: 3 in]
        n593 = call "Convert to Dynamic Data5"("Array"=w830) -> ("Dynamic Data Type"=w895:dynamicdata)  [unwired: 3 in]
        n594 = call "Convert to Dynamic Data6"("Array"=w829) -> ("Dynamic Data Type"=w894:dynamicdata)  [unwired: 3 in]
        n595 = call "Convert to Dynamic Data7"("Array"=w828) -> ("Dynamic Data Type"=w893:dynamicdata)  [unwired: 3 in]
        n596 = call "Convert to Dynamic Data8"("Array"=w827) -> ("Dynamic Data Type"=w892:dynamicdata)  [unwired: 3 in]
        n597 = call "Convert to Dynamic Data9"("Array"=w826) -> ("Dynamic Data Type"=w891:dynamicdata)  [unwired: 3 in]
        n598 = call "Convert to Dynamic Data10"("Array"=w825) -> ("Dynamic Data Type"=w890:dynamicdata)  [unwired: 3 in]
        n599 = call "Convert to Dynamic Data11"("Array"=w824) -> ("Dynamic Data Type"=w889:dynamicdata)  [unwired: 3 in]
        n600 = call "Convert to Dynamic Data12"("Array"=w823) -> ("Dynamic Data Type"=w888:dynamicdata)  [unwired: 3 in]
        n601 = call "Convert to Dynamic Data13"("Array"=w822) -> ("Dynamic Data Type"=w887:dynamicdata)  [unwired: 3 in]
        n602 = call "Convert to Dynamic Data14"("Array"=w821) -> ("Dynamic Data Type"=w886:dynamicdata)  [unwired: 3 in]
        n603 = call "Convert to Dynamic Data15"("Array"=w820) -> ("Dynamic Data Type"=w885:dynamicdata)  [unwired: 3 in]
        n604 = call "Convert to Dynamic Data16"("Array"=w819) -> ("Dynamic Data Type"=w884:dynamicdata)  [unwired: 3 in]
        n605 = call "Convert to Dynamic Data33"("Array"=w818) -> ("Dynamic Data Type"=w883:dynamicdata)  [unwired: 3 in]
        n606 = call "Convert to Dynamic Data34"("Array"=w817) -> ("Dynamic Data Type"=w882:dynamicdata)  [unwired: 3 in]
        n607 = call "Convert to Dynamic Data35"("Array"=w816) -> ("Dynamic Data Type"=w881:dynamicdata)  [unwired: 3 in]
        n608 = call "Convert to Dynamic Data36"("Array"=w815) -> ("Dynamic Data Type"=w880:dynamicdata)  [unwired: 3 in]
        n609 = call "Convert to Dynamic Data37"("Array"=w814) -> ("Dynamic Data Type"=w879:dynamicdata)  [unwired: 3 in]
        n610 = call "Convert to Dynamic Data38"("Array"=w813) -> ("Dynamic Data Type"=w878:dynamicdata)  [unwired: 3 in]
        n611 = call "Convert to Dynamic Data39"("Array"=w812) -> ("Dynamic Data Type"=w877:dynamicdata)  [unwired: 3 in]
        n612 = call "Convert to Dynamic Data40"("Array"=w811) -> ("Dynamic Data Type"=w876:dynamicdata)  [unwired: 3 in]
        n613 = call "Convert to Dynamic Data41"("Array"=w810) -> ("Dynamic Data Type"=w875:dynamicdata)  [unwired: 3 in]
        n614 = call "Convert to Dynamic Data42"("Array"=w809) -> ("Dynamic Data Type"=w874:dynamicdata)  [unwired: 3 in]
        n615 = call "Convert to Dynamic Data43"("Array"=w808) -> ("Dynamic Data Type"=w873:dynamicdata)  [unwired: 3 in]
        n616 = call "Convert to Dynamic Data44"("Array"=w807) -> ("Dynamic Data Type"=w872:dynamicdata)  [unwired: 3 in]
        n617 = call "Convert to Dynamic Data45"("Array"=w806) -> ("Dynamic Data Type"=w871:dynamicdata)  [unwired: 3 in]
        n618 = call "Convert to Dynamic Data46"("Array"=w805) -> ("Dynamic Data Type"=w870:dynamicdata)  [unwired: 3 in]
        n619 = call "Convert to Dynamic Data47"("Array"=w804) -> ("Dynamic Data Type"=w869:dynamicdata)  [unwired: 3 in]
        n620 = call "Convert to Dynamic Data48"("Array"=w803) -> ("Dynamic Data Type"=w868:dynamicdata)  [unwired: 3 in]
        n621 = call <vilib>:"Std Deviation and Variance.vi"("X"=w834, "Weighting (Sample)"=w835) -> ("mean"=w982:dbl, "standard deviation"=w981:dbl)  [unwired: 1 out]
        n622 = call <vilib>:"Std Deviation and Variance.vi"("X"=w833, "Weighting (Sample)"=w835) -> ("mean"=w980:dbl, "standard deviation"=w979:dbl)  [unwired: 1 out]
        n623 = call <vilib>:"Std Deviation and Variance.vi"("X"=w832, "Weighting (Sample)"=w835) -> ("mean"=w978:dbl, "standard deviation"=w977:dbl)  [unwired: 1 out]
        n624 = call <vilib>:"Std Deviation and Variance.vi"("X"=w831, "Weighting (Sample)"=w835) -> ("mean"=w976:dbl, "standard deviation"=w975:dbl)  [unwired: 1 out]
        n625 = call <vilib>:"Std Deviation and Variance.vi"("X"=w830, "Weighting (Sample)"=w835) -> ("mean"=w974:dbl, "standard deviation"=w973:dbl)  [unwired: 1 out]
        n626 = call <vilib>:"Std Deviation and Variance.vi"("X"=w829, "Weighting (Sample)"=w835) -> ("mean"=w971:dbl, "standard deviation"=w967:dbl)  [unwired: 1 out]
        n627 = call <vilib>:"Std Deviation and Variance.vi"("X"=w828, "Weighting (Sample)"=w835) -> ("mean"=w972:dbl, "standard deviation"=w966:dbl)  [unwired: 1 out]
        n628 = call <vilib>:"Std Deviation and Variance.vi"("X"=w827, "Weighting (Sample)"=w835) -> ("mean"=w970:dbl, "standard deviation"=w965:dbl)  [unwired: 1 out]
        n629 = call <vilib>:"Std Deviation and Variance.vi"("X"=w826, "Weighting (Sample)"=w835) -> ("mean"=w969:dbl, "standard deviation"=w964:dbl)  [unwired: 1 out]
        n630 = call <vilib>:"Std Deviation and Variance.vi"("X"=w825, "Weighting (Sample)"=w835) -> ("mean"=w968:dbl, "standard deviation"=w963:dbl)  [unwired: 1 out]
        n631 = call <vilib>:"Std Deviation and Variance.vi"("X"=w824, "Weighting (Sample)"=w835) -> ("mean"=w962:dbl, "standard deviation"=w951:dbl)  [unwired: 1 out]
        n632 = call <vilib>:"Std Deviation and Variance.vi"("X"=w823, "Weighting (Sample)"=w835) -> ("mean"=w961:dbl, "standard deviation"=w952:dbl)  [unwired: 1 out]
        n633 = call <vilib>:"Std Deviation and Variance.vi"("X"=w822, "Weighting (Sample)"=w835) -> ("mean"=w960:dbl, "standard deviation"=w953:dbl)  [unwired: 1 out]
        n634 = call <vilib>:"Std Deviation and Variance.vi"("X"=w821, "Weighting (Sample)"=w835) -> ("mean"=w959:dbl, "standard deviation"=w954:dbl)  [unwired: 1 out]
        n635 = call <vilib>:"Std Deviation and Variance.vi"("X"=w820, "Weighting (Sample)"=w835) -> ("mean"=w958:dbl, "standard deviation"=w955:dbl)  [unwired: 1 out]
        n636 = call <vilib>:"Std Deviation and Variance.vi"("X"=w819, "Weighting (Sample)"=w835) -> ("mean"=w957:dbl, "standard deviation"=w956:dbl)  [unwired: 1 out]
        n637 = call <vilib>:"Std Deviation and Variance.vi"("X"=w818, "Weighting (Sample)"=w835) -> ("mean"=w867:dbl, "standard deviation"=w866:dbl)  [unwired: 1 out]
        n638 = call <vilib>:"Std Deviation and Variance.vi"("X"=w817, "Weighting (Sample)"=w835) -> ("mean"=w865:dbl, "standard deviation"=w864:dbl)  [unwired: 1 out]
        n639 = call <vilib>:"Std Deviation and Variance.vi"("X"=w816, "Weighting (Sample)"=w835) -> ("mean"=w863:dbl, "standard deviation"=w862:dbl)  [unwired: 1 out]
        n640 = call <vilib>:"Std Deviation and Variance.vi"("X"=w815, "Weighting (Sample)"=w835) -> ("mean"=w861:dbl, "standard deviation"=w860:dbl)  [unwired: 1 out]
        n641 = call <vilib>:"Std Deviation and Variance.vi"("X"=w814, "Weighting (Sample)"=w835) -> ("mean"=w859:dbl, "standard deviation"=w858:dbl)  [unwired: 1 out]
        n642 = call <vilib>:"Std Deviation and Variance.vi"("X"=w813, "Weighting (Sample)"=w835) -> ("mean"=w856:dbl, "standard deviation"=w852:dbl)  [unwired: 1 out]
        n643 = call <vilib>:"Std Deviation and Variance.vi"("X"=w812, "Weighting (Sample)"=w835) -> ("mean"=w857:dbl, "standard deviation"=w851:dbl)  [unwired: 1 out]
        n644 = call <vilib>:"Std Deviation and Variance.vi"("X"=w811, "Weighting (Sample)"=w835) -> ("mean"=w855:dbl, "standard deviation"=w850:dbl)  [unwired: 1 out]
        n645 = call <vilib>:"Std Deviation and Variance.vi"("X"=w810, "Weighting (Sample)"=w835) -> ("mean"=w854:dbl, "standard deviation"=w849:dbl)  [unwired: 1 out]
        n646 = call <vilib>:"Std Deviation and Variance.vi"("X"=w809, "Weighting (Sample)"=w835) -> ("mean"=w853:dbl, "standard deviation"=w848:dbl)  [unwired: 1 out]
        n647 = call <vilib>:"Std Deviation and Variance.vi"("X"=w808, "Weighting (Sample)"=w835) -> ("mean"=w847:dbl, "standard deviation"=w836:dbl)  [unwired: 1 out]
        n648 = call <vilib>:"Std Deviation and Variance.vi"("X"=w807, "Weighting (Sample)"=w835) -> ("mean"=w846:dbl, "standard deviation"=w837:dbl)  [unwired: 1 out]
        n649 = call <vilib>:"Std Deviation and Variance.vi"("X"=w806, "Weighting (Sample)"=w835) -> ("mean"=w845:dbl, "standard deviation"=w838:dbl)  [unwired: 1 out]
        n650 = call <vilib>:"Std Deviation and Variance.vi"("X"=w805, "Weighting (Sample)"=w835) -> ("mean"=w844:dbl, "standard deviation"=w839:dbl)  [unwired: 1 out]
        n651 = call <vilib>:"Std Deviation and Variance.vi"("X"=w804, "Weighting (Sample)"=w835) -> ("mean"=w843:dbl, "standard deviation"=w840:dbl)  [unwired: 1 out]
        n652 = call <vilib>:"Std Deviation and Variance.vi"("X"=w803, "Weighting (Sample)"=w835) -> ("mean"=w842:dbl, "standard deviation"=w841:dbl)  [unwired: 1 out]
        n653 = Merge Signals(w899, w898, w897, w896, w895, w894, w893, w892, w891, w890, w889, w888, w887, w886, w885, w884, w883, w882, w881, w880, w879, w878, w877, w876, w875, w874, w873, w872, w871, w870, w869, w868) -> (w987:dynamicdata)
        n654 = Build Array(w982, w981) -> (w802:dbl[])
        n655 = Build Array(w980, w979) -> (w800:dbl[])
        n656 = Build Array(w978, w977) -> (w798:dbl[])
        n657 = Build Array(w976, w975) -> (w796:dbl[])
        n658 = Build Array(w974, w973) -> (w794:dbl[])
        n659 = Build Array(w971, w967) -> (w792:dbl[])
        n660 = Build Array(w972, w966) -> (w790:dbl[])
        n661 = Build Array(w970, w965) -> (w788:dbl[])
        n662 = Build Array(w969, w964) -> (w786:dbl[])
        n663 = Build Array(w968, w963) -> (w784:dbl[])
        n664 = Build Array(w962, w951) -> (w782:dbl[])
        n665 = Build Array(w961, w952) -> (w780:dbl[])
        n666 = Build Array(w960, w953) -> (w778:dbl[])
        n667 = Build Array(w959, w954) -> (w776:dbl[])
        n668 = Build Array(w958, w955) -> (w774:dbl[])
        n669 = Build Array(w957, w956) -> (w772:dbl[])
        n670 = Build Array(w867, w866) -> (w770:dbl[])
        n671 = Build Array(w865, w864) -> (w768:dbl[])
        n672 = Build Array(w863, w862) -> (w766:dbl[])
        n673 = Build Array(w861, w860) -> (w764:dbl[])
        n674 = Build Array(w859, w858) -> (w762:dbl[])
        n675 = Build Array(w856, w852) -> (w760:dbl[])
        n676 = Build Array(w857, w851) -> (w758:dbl[])
        n677 = Build Array(w855, w850) -> (w756:dbl[])
        n678 = Build Array(w854, w849) -> (w754:dbl[])
        n679 = Build Array(w853, w848) -> (w752:dbl[])
        n680 = Build Array(w847, w836) -> (w750:dbl[])
        n681 = Build Array(w846, w837) -> (w748:dbl[])
        n682 = Build Array(w845, w838) -> (w746:dbl[])
        n683 = Build Array(w844, w839) -> (w744:dbl[])
        n684 = Build Array(w843, w840) -> (w742:dbl[])
        n685 = Build Array(w842, w841) -> (w740:dbl[])
        n686 = local read "appended array"() -> (w991:string[])
        n687 = call "Convert to Dynamic Data17"("Array"=w802) -> ("Dynamic Data Type"=w801:dynamicdata)  [unwired: 3 in]
        n688 = call "Convert to Dynamic Data18"("Array"=w800) -> ("Dynamic Data Type"=w799:dynamicdata)  [unwired: 3 in]
        n689 = call "Convert to Dynamic Data19"("Array"=w798) -> ("Dynamic Data Type"=w797:dynamicdata)  [unwired: 3 in]
        n690 = call "Convert to Dynamic Data20"("Array"=w796) -> ("Dynamic Data Type"=w795:dynamicdata)  [unwired: 3 in]
        n691 = call "Convert to Dynamic Data21"("Array"=w794) -> ("Dynamic Data Type"=w793:dynamicdata)  [unwired: 3 in]
        n692 = call "Convert to Dynamic Data22"("Array"=w792) -> ("Dynamic Data Type"=w791:dynamicdata)  [unwired: 3 in]
        n693 = call "Convert to Dynamic Data23"("Array"=w790) -> ("Dynamic Data Type"=w789:dynamicdata)  [unwired: 3 in]
        n694 = call "Convert to Dynamic Data24"("Array"=w788) -> ("Dynamic Data Type"=w787:dynamicdata)  [unwired: 3 in]
        n695 = call "Convert to Dynamic Data25"("Array"=w786) -> ("Dynamic Data Type"=w785:dynamicdata)  [unwired: 3 in]
        n696 = call "Convert to Dynamic Data26"("Array"=w784) -> ("Dynamic Data Type"=w783:dynamicdata)  [unwired: 3 in]
        n697 = call "Convert to Dynamic Data27"("Array"=w782) -> ("Dynamic Data Type"=w781:dynamicdata)  [unwired: 3 in]
        n698 = call "Convert to Dynamic Data28"("Array"=w780) -> ("Dynamic Data Type"=w779:dynamicdata)  [unwired: 3 in]
        n699 = call "Convert to Dynamic Data29"("Array"=w778) -> ("Dynamic Data Type"=w777:dynamicdata)  [unwired: 3 in]
        n700 = call "Convert to Dynamic Data30"("Array"=w776) -> ("Dynamic Data Type"=w775:dynamicdata)  [unwired: 3 in]
        n701 = call "Convert to Dynamic Data31"("Array"=w774) -> ("Dynamic Data Type"=w773:dynamicdata)  [unwired: 3 in]
        n702 = call "Convert to Dynamic Data32"("Array"=w772) -> ("Dynamic Data Type"=w771:dynamicdata)  [unwired: 3 in]
        n703 = call "Convert to Dynamic Data49"("Array"=w770) -> ("Dynamic Data Type"=w769:dynamicdata)  [unwired: 3 in]
        n704 = call "Convert to Dynamic Data50"("Array"=w768) -> ("Dynamic Data Type"=w767:dynamicdata)  [unwired: 3 in]
        n705 = call "Convert to Dynamic Data51"("Array"=w766) -> ("Dynamic Data Type"=w765:dynamicdata)  [unwired: 3 in]
        n706 = call "Convert to Dynamic Data52"("Array"=w764) -> ("Dynamic Data Type"=w763:dynamicdata)  [unwired: 3 in]
        n707 = call "Convert to Dynamic Data53"("Array"=w762) -> ("Dynamic Data Type"=w761:dynamicdata)  [unwired: 3 in]
        n708 = call "Convert to Dynamic Data54"("Array"=w760) -> ("Dynamic Data Type"=w759:dynamicdata)  [unwired: 3 in]
        n709 = call "Convert to Dynamic Data55"("Array"=w758) -> ("Dynamic Data Type"=w757:dynamicdata)  [unwired: 3 in]
        n710 = call "Convert to Dynamic Data56"("Array"=w756) -> ("Dynamic Data Type"=w755:dynamicdata)  [unwired: 3 in]
        n711 = call "Convert to Dynamic Data57"("Array"=w754) -> ("Dynamic Data Type"=w753:dynamicdata)  [unwired: 3 in]
        n712 = call "Convert to Dynamic Data58"("Array"=w752) -> ("Dynamic Data Type"=w751:dynamicdata)  [unwired: 3 in]
        n713 = call "Convert to Dynamic Data59"("Array"=w750) -> ("Dynamic Data Type"=w749:dynamicdata)  [unwired: 3 in]
        n714 = call "Convert to Dynamic Data60"("Array"=w748) -> ("Dynamic Data Type"=w747:dynamicdata)  [unwired: 3 in]
        n715 = call "Convert to Dynamic Data61"("Array"=w746) -> ("Dynamic Data Type"=w745:dynamicdata)  [unwired: 3 in]
        n716 = call "Convert to Dynamic Data62"("Array"=w744) -> ("Dynamic Data Type"=w743:dynamicdata)  [unwired: 3 in]
        n717 = call "Convert to Dynamic Data63"("Array"=w742) -> ("Dynamic Data Type"=w741:dynamicdata)  [unwired: 3 in]
        n718 = call "Convert to Dynamic Data64"("Array"=w740) -> ("Dynamic Data Type"=w739:dynamicdata)  [unwired: 3 in]
        n719 = Merge Signals(w801, w799, w797, w795, w793, w791, w789, w787, w785, w783, w781, w779, w777, w775, w773, w771, w769, w767, w765, w763, w761, w759, w757, w755, w753, w751, w749, w747, w745, w743, w741, w739) -> (w986:dynamicdata)
        n720 = Select(t=w987, s="Datapath", f=w986) -> (s? t:f=w985:dynamicdata)
        n721 = TDMS Write(0:w989, 1:enum16{"decimated", "interleaved"}."decimated" ("data layout (0:decimated)"), 5:"Mediciones USB-6009" ("group name in (Untitled)"), 7:w991, 9:w985) -> ()  [unwired: 1 in, 4 out]
        n722 = property on="Guardar" class="Bool (strict)"("Value"=FALSE ("Boolean 18")) -> ()  [unwired: 2 in, 2 out]
      }
    }
    n723 = property on="Boolean 10" class="Bool (strict)"() -> ("Value"=w643:bool)  [unwired: 2 in, 2 out]
    "CH1" <- "CH1"
    "CH2" <- "CH2 2"
    "CH3" <- "CH3"
    "CH4" <- "CH4 2"
    "CH5" <- "CH5"
    "CH6" <- "CH6"
    "CH7" <- "CH7"
    "CH8" <- "CH8"
    "Boolean 9" <- "Iniciar"
    "CH1" <- "CH1"
    "CH2" <- "CH2 2"
    "CH3" <- "CH3"
    "CH4" <- "CH4 2"
    "CH5" <- "CH5"
    "CH6" <- "CH6"
    "CH7" <- "CH7"
    "CH8" <- "CH8"
    "CH9" <- "CH9"
    "CH9 3" <- "CH9"
    "CH10 2" <- "CH10"
    "CH11 2" <- "CH11"
    "CH12 2" <- "CH12"
    "CH13 2" <- "CH13"
    "CH14 2" <- "CH14"
    "CH15 2" <- "CH15"
    "CH16 2" <- "CH16"
    "CH10" <- "CH10"
    "CH11" <- "CH11"
    "CH12" <- "CH12"
    "CH13 3" <- "CH13"
    "CH14 3" <- "CH14"
    "CH15 3" <- "CH15"
    "CH16 3" <- "CH16"
  }
  n724 = property on="b13" class="DigNum (strict)"("Value"=w14) -> ()  [unwired: 2 in, 2 out]
  n725 = call-poly <vilib>:"Read Key.vi"("section"=w6, "error in (no error)"=w16, "key"="B14", "refnum"=w17) -> ("error out"=w11:errorcluster, "value"=w5:dbl, "refnum out"=w10:T4)  [unwired: 4 in, 1 out]
  n726 = property on="b14" class="DigNum (strict)"("Value"=w5) -> ()  [unwired: 2 in, 2 out]
  n727 = call-poly <vilib>:"Read Key.vi"("section"=w6, "error in (no error)"=w11, "key"="B15", "refnum"=w10) -> ("error out"=w8:errorcluster, "value"=w4:dbl, "refnum out"=w7:T4)  [unwired: 4 in, 1 out]
  n728 = property on="b15" class="DigNum (strict)"("Value"=w4) -> ()  [unwired: 2 in, 2 out]
  n729 = call-poly <vilib>:"Read Key.vi"("section"=w6, "error in (no error)"=w8, "key"="B16", "refnum"=w7) -> ("error out"=w2:errorcluster, "value"=w1:dbl, "refnum out"=w3:T4)  [unwired: 4 in, 1 out]
  n730 = property on="b16" class="DigNum (strict)"("Value"=w1) -> ()  [unwired: 2 in, 2 out]
  n731 = call <vilib>:"Close Config Data.vi"("error in (no error)"=w2, "refnum"=w3) -> ()  [unwired: 8 in, 2 out]
